vi "MAIN - PECT - Autonics - Pulses.vi"() -> ()   [LabVIEW 2018]
uses:
  Control 1.ctl
  <vilib>/DAQmx/read.llb/DAQmx Read (Counter U32 1Chan 1Samp).vi
  <vilib>/DAQmx/write.llb/DAQmx Write (Analog 1D Wfm NChan NSamp).vi
  <vilib>/DAQmx/read.llb/DAQmx Read (Analog 1D Wfm NChan NSamp).vi
  <vilib>/Instr/_visa.llb/VISA Configure Serial Port (Instr).vi
  <vilib>/DAQmx/create/channels.llb/DAQmx Create Channel (AI-Voltage-Basic).vi
  <vilib>/DAQmx/create/channels.llb/DAQmx Create Channel (CI-Count Edges).vi
  <vilib>/DAQmx/miscellaneous.llb/DAQmx Fill In Error Info.vi
  <vilib>/DAQmx/configure/timing.llb/DAQmx Timing (Sample Clock).vi
  <vilib>/DAQmx/configure/trigger.llb/DAQmx Start Trigger (Digital Edge).vi
  <vilib>/DAQmx/create/channels.llb/DAQmx Create Channel (AO-Voltage-Basic).vi
  Global_data.vi
  <vilib>/express/express analysis/Spectral/Block/exnSpectralBlock spectral measurements PSD poly.vi
  <vilib>/express/express analysis/Spectral/Block/exnSpectralBlock spectral measurements PSD WFM.vi
  <vilib>/express/express analysis/Spectral/XNode/ExpressSpectralMeasurementsBlockNode.xnode
  <resource>/objmgr/daqmx.rc
  <vilib>/Platform/NI_3dgraph.lvlib
panel:
  out "x <= y?":bool
  in  "Motor counter":tag="Dev3/ctr0"
  in  "Motor Counter Terminal":tag="PFI8"
  out "dy":dbl[][](array[numeric])=[[0.02185273217949213, 0.22162137391350623, 0.3780063347527216, 0.47366728119120083, 0.5155987387622605, 0.5344849660156372, 0.5340327156552669, 0.5179164395979683, 0.4924534388561326, 0.4657014009743683, 0.4395619065458265, 0.41345477245652273, 0.38299660763801213, 0.35485913243808975, 0.32430442308230173, 0.30445032009464046, 0.27550721525097666, 0.251882180054519, 0.23418758796048045, 0.2142368598869009, 0.19357706032981925, 0.1801369179101573, 0.1648273984200661, 0.15686645912775665, 0.13830164031007763, 0.12063927272359809, 0.11206594020999994, 0.10861727814154509, 0.09356558004140059, 0.0861847728629872, 0.07722466077804135, 0.07770813065864868, 0.0689091681320213, 0.06265642589408449, 0.055372300069219005, 0.052600467323083766, 0.0475402553312021, 0.041770966987191294, 0.037323135461628354, 0.039031364875901975, 0.03471245509778598, 0.03148938809455126, 0.028782011620806625, 0.02665478726769166, 0.026268020417924642, 0.021852415607831688, 0.014922815304144965, 0.020015267194226194, 0.01804919503626312, 0.01572858483151185, 0.014568279890680547, 0.01592197018079, 0.018564888990501682, 0.01208651666644922, 0.006156065869896921, 0.008379985211604435, 0.012924516058780533, 0.006703988431595143, 0.006865142169170113, 0.005285837275303962, 0.011377442504307389, 0.008412216926839022, 0.006220528313659379, 0.006800681356610383, 0.0037065325418499384, 0.005801529216698853, 0.0029329953769190453, 0.0017726895292300426, 0.006639528072359013, 0.006188298098165568, 0.002997456934826559, 0.0038354556699644604, 0.004673454442502667, 0.005124684635743115, 0.0007735372999029266, -0.00029007654728996357, 0.0031263799247724933, 0.003996609454210542, 0.0011925366909029123, 0.0018693819072517215, 0.0036098409046472213, 0.008122142002352284, 0.0008702294956277612, -0.001095844667359458, -0.001418151804670309, 0.0045445320082038165, 0.0010313830870058993, 0.0007413066156765069, -0.0022239198542619576, 0.008379987983489379, 0.0013536903608795114, -0.0002578458337252343, 0.0016115362047441906, 0.001901612692167376, -0.0004834608665751361, 0.0008379988404314531, -0.0008702295433602458, 0.003319764541380721, 0.0022239199677400734, 0.0014503825811269522, -0.0015148440421395293, 0.0035131489465634047, 0.0017404591631580146, -0.0021594585229163243, -0.0020627664120063116, 0.0014503825799989656, 0.0022883814364993427, 0.002030535662503219, -0.001063613882371861, 0.0025462272945091513, 0.007155221045837656, -0.0023206122806760376, -0.002771842462127694, -0.00077353738382957, -0.00022561499425499676, 0.0016759976704383561, 0.0009669217607966019, -0.004608993606950662, 0.0077676047046848495, 0.0011925368038836481, -0.0016115363216133716, 0.0007413066839978555, 0.0002578458568640585, -0.00035453803645157933, -0.00273961161100722, 0.0020305356825334187, 0.0021594585699595825, 0.0021272279138271344, -0.0003223072593838694, -0.0014503826419236532, 0.002900765285667184, 0.0005801531028586382, -0.0023528429885493196, -0.0019660742882070537, 0.00032230723191783994, 0.002385073698162543, 0.0020305357420138392, -0.0010313832066026762, 0.0011925368768670452, 0.008057681666933547, -0.003964379420267505, -0.004254455948108138, -0.0006768452007133163, 0.001998305074122797, -0.0017082284897318445, 0.0013859212221971617, -0.0032553032595314946, 0.006123837900990026, -9.669220003782897e-05, -0.0004834609598374229, -0.0012247676106964533, 0.0010958447384830095, -0.0006768452835217431, -0.0022561507887344234, 0.0010636139879691697, 0.004286686496722147, 0.0010958447184945541, 3.22307075428796e-05, -0.002610688825346763, 0.003255303372588614, -0.00029007653819057566, -0.0038676871668865687, -0.0012569982994836693, 0.0027073809723914266, 0.0008379988720914611, 0.001837151388540903, -0.0011603061375105028, 0.00022561513089769392, 0.005350300672845698, -0.0019016129023885497, -0.0032875342027223198, -0.0015470748241881438, 0.0013859212779196994, 9.669220112495935e-05, -0.0008379989032860635, -0.00022561506580132118, 0.004286686619572322, 0.00022561507642038237, -0.0023528431049744114, -0.0006123838295124528, 0.0008379989115052666, -0.0006768452570238281, -0.0020949971695305436, 0.001675997810987262, 0.0032875340175193557, 0.000999152537735526, 9.669215431618028e-05, -0.0019983050408773906, 0.0012569983738517365, 0.0005801530509979003, -0.0033197648624758713, -0.001933843537593738, 0.0023528430139325707, 0.002352843003613714, 3.2230727526005865e-05, 0.0003867687163454647, 0.00019338437490290517, 0.004254456017976693, -0.0032230727316582275, -0.0020949972828692154, -0.0008702296034401868, 0.0013859212870555027, -0.0002900765149931317, 0.0004189994079704107, -0.0018371514061916727, 0.004512301822965803, -0.0007735374888504509, -0.0014503827796508162, -0.0009024603734397729, 0.0011603061884652988, -0.001611536337480679, -0.002159458641943779, 0.0015148441911065902, 0.004770147471044872, -6.446143959504269e-05, -0.00012892292785871007, -0.0019660743144251924, 0.002223920178802352, -0.0020627665501065096, -0.00119253690483756, -0.0020949971905164233, 0.001998305023551694, 0.000837998893217673, 0.0011925368763803235, -0.0009346910904382, 0.002127227990854408, 0.0019660744327474333, -0.0017404593293584014, -0.0027718425051004303, -0.0011603061738929554, 0.0011603061928742164, 3.223074204505849e-05, -0.00019338439914129424, 0.0006123838137348514, 0.0024817660569604882, 0.00012892286886057036, -0.0007090760386532224, -0.000225615129568979, -0.00016115363443436337, -0.0006123837841736091, -0.0024495352188536046, 0.0014826134650398615, 0.0032875340681286502, 0.0008057681913156145, -0.0017082285571126121, -0.0007413066611023922, 0.0020627665464481026, -0.000999152585484886, -0.002256150873965801, -0.012408829591370463, -0.021433432067929914, -0.22197293874851098, -0.3764222806586943, -0.46740915295030705, -0.5164638338272902, -0.5334490578309308, -0.5352859904035077, -0.5179780628156556, -0.4965124995471779, -0.46740836721638884, -0.4402703575389572, -0.41110184791818216, -0.3806441179057998, -0.35328052056021786, -0.3275928987712948, -0.3012284032192838, -0.2752506398248955, -0.25397853054603514, -0.23493031326555158, -0.21491513953837904, -0.1958023955316519, -0.17643177172610525, -0.16411968228431473, -0.15132410993446976, -0.13846405632706293, -0.1227998907450889, -0.11590252592732764, -0.10665229070022342, -0.09727311992830856, -0.08679808396375766, -0.08019075848337298, -0.07368011952376108, -0.06742732255462158, -0.06049766823168046, -0.05608203042605808, -0.053213480482009246, -0.0475730563911565, -0.043705337617349294, -0.04022438977457732, -0.037935990066018555, -0.03374595466774899, -0.030458387820377908, -0.028621219564915812, -0.026203890291860432, -0.025752658006232387, -0.019467593462318078, -0.01927420876953434, -0.02078907336652236, -0.020176684123793365, -0.015567634743558045, -0.013246994438153692, -0.013118070851520613, -0.014407317066149616, -0.013537077661091246, -0.009347030152641267, -0.010668507561701013, -0.009798267022355311, -0.010088347912076578, -0.008090017555329787, -0.007445394773112568, -0.00928257069176297, -0.005092521345138934, -0.0058338382012763645, -0.004125587253031249, -0.00728424031063124, -0.005028059898926074, -0.0032231152560280307, -0.005801607890615124, -0.005092522415750089, -0.005801608187410601, -0.0037065829285172214, -0.002320643368463493, -0.004834673724378291, -0.0028041107197980253, -0.0015148644444460402, -0.00022561814109067768, -0.00409335720323778, -0.00438343776733241, -0.0029974979706475224, -0.0009024725041406612, -0.003384271962996621, -0.002449568288255044, -0.0026751867248657746, 0.0009024725590478511, -0.00286857347007885, -0.0007090853837512512, -0.0033198098144016086, -0.0010958596788803732, -0.0028041112816303837, -0.0018694075623315598, -0.0011603217624793771, 3.223115459860537e-05, -0.00016115582712750154, -0.0013537089395612156, -0.003480965935072966, 0.0026429556728508885, -0.003061960775959882, -0.000870241426966345, -0.004737981658807122, 0.0011925533678454059, -0.0014826337024933522, -0.00038677395914277213, -0.001933870000138782, 0.0021594881681208378, 0.0010636284382137262, -0.001998332242745704, -0.002836342690361704, -0.002965267523460824, 0.001321477918626357, -0.00025784932654815407, -0.003287579153148812, -3.223132886898128e-05, 0.0026107244517081796, -0.00012892453675217297, -0.0013859400535904953, -0.0014504025112538343, -6.4462473896576e-05, -0.0030941922480201, -0.0012247844018435927, -0.00016115567855923274, 0.002127257150072559, 0.0013537090959196973, -0.0016760207747053002, -0.0017082520566722437, 0.0023206442516912063, -0.002127257163786034, -0.0019983324466084085, -0.0012570157816984562, -0.0010958596522536723, 0.0020627948594293954, 0.000419005267335848, -0.002900805281237595, 0.002739649366902519, 0.0035454285251645956, -0.00438343887530479, -0.0011280909248192472, -0.003061961217107445, 0.0024495689780037466, -3.223119648865236e-05, -0.0016760208118133946, -0.0010636287683363221, 0.0033520414134819987, -0.0004190049852823563, -0.0026429558725240554, -0.0011925531630785358, 0.0015470960247538912, -0.0027074183199484736, -0.001289246809195177, 0.00128924691794019, 0.002610724760119254, 0.001901639043667025, -0.0030941922624947438, -0.0032231171698793304, 0.0060272289191773964, -0.004931368989611329, -0.0008702416052575046, -0.0019016393047914804, 0.0020305639428972455, 0.0012892468470901974, 0.0006446234421115804, -0.002610724837572853, 0.0019016390284969376, 0.0015793272920747725, -0.0017082519598439205, -0.002900805364877357, -0.000709085817734767, 0.0028041119282748994, -0.00016115587107901064, -0.0018049455564170813, 0.00022561808799004268, 0.0013537090055955048, 0.0008380105330507703, -0.003255348141158798, -0.00035454279478663864, 0.0018371766375260279, -0.0035776600751207255, -0.0004190052285268919, 0.002900805448792454, 0.002223950819624676, 0.0018694079109380368, -0.0032553481382180394, -0.0032875795671039043, 0.004447901674611288, -0.0025784936590147467, -0.0016115585622911155, -0.002127257495139645, 0.003255348419116011, 0.0018371768337592798, -0.001128090974523488, -0.0009669351580914309, 0.0009024727918127695, 0.001128090987530861, -0.0025140313757301413, -0.0011603221493157179, -0.0009669351707461971, 0.0036743535752394862, -0.0016437897422942882, -0.00016115587246545715, -0.0003867741019458748, 0.00077354797094209, 0.0001289246734081928, -0.0019338701466384833, -0.0028363430810758317, 0.004351208139382834, -0.003029730220318605, -0.00048346763104412105, 0.0020627950775606863, 0.004415670395760962, 0.0001933871398263065, -0.0042867457023128, -0.0020305639252988783, 0.004351208217657998, -0.0028685742179446194, -0.000966935188323248, -0.003932203230262665, 0.005833842290003943, 0.001676021002762873, -0.0002578493208744703, -0.0023528755324573325, 0.0001933869506860475, -0.0015793273811111064, 0.0009024727892432693, -0.0025784937121944296, 0.0008057793101148292, 0.005608223865920969, -0.0019983326508024035, -0.0013859403391727199, 0.0009991662564088344, 0.000386773835537646, -0.0011280909016528895, -0.0028685742308987017, -0.001063628580464382, 0.0019016390821331441, 0.000451236446354919, -0.0012247846328268253, 0.002127257322039, 0.005060293783419212, -0.0009347038394702523, -0.005350374306660299, -0.000322311809180853, 0.00228841316574524, -0.0023528754941306573, -0.0006446235024473168, -0.0026751874774042506, 0.005092525334164044, 0.004028896469372434, -0.004770213274351676, -0.0007413169580825496, 0.0015470961610528633], [0.026784100031834512, 0.22565025518823933, 0.3745898180588192, 0.4658351284321114, 0.5195309092491112, 0.5352584960489501, 0.5372235546955544, 0.5137586578368909, 0.49219558678815245, 0.4708260749714661, 0.4421403513412341, 0.41177877159702825, 0.37458440957515166, 0.35463351738372256, 0.3285910937384298, 0.29984134272168944, 0.27844020024186034, 0.24917480927999724, 0.2327049801329557, 0.21581615988325065, 0.19805711606493515, 0.1764948588357853, 0.15873581094289735, 0.15038810220007237, 0.13901071275952415, 0.12424910299364411, 0.11619146185751328, 0.09917369791631492, 0.09872248304086018, 0.08898883938039681, 0.08389640742510363, 0.0708752299975064, 0.0624952645947654, 0.06462249593467728, 0.058144137574782206, 0.054566538291412225, 0.0439304186397127, 0.04270565633641521, 0.04160981659824259, 0.03767767582517134, 0.03825783118913595, 0.02359286790303816, 0.027911782375556804, 0.02868532082928832, 0.025268868363350627, 0.02265818289102217, 0.016276504724094476, 0.019112807239303642, 0.01946734585367027, 0.016340968153478297, 0.01701781357957932, 0.0065428338386475104, 0.012924514293859879, 0.015019510914417111, 0.011280748870691415, 0.010990672788820266, 0.005865989716593134, 0.010700596721945121, 0.010700597051142235, 0.01024936728566983, 0.00667175803059461, 0.0016759972379327692, 0.00818660189065934, 0.007993217768344607, 0.009443600123263174, -2.8045121780451154e-11, 0.0060271442455350765, 0.006317220804501922, 0.005092453598039448, 0.0069940660319938175, -0.0012247673040803875, 0.0008057679314195099, 0.004770146517182106, 0.006381682601488414, 0.004318916540771767, -0.0033519948913074415, 0.003642071348493481, 0.004028840109692844, 0.0029007649154300097, 0.003319764295098615, -0.0015148438851326773, -0.0002900765221385271, 0.004061070905809316, 0.0037065330108747574, 0.002707380653014013, -0.0028685342311973727, 0.003835455906583185, 0.005124684906207655, 0.003609840897486727, -6.446145531402436e-05, -0.0012569981537113861, 0.001514844018148942, 0.0026429193096486614, 0.006671759686645906, -0.002578457828548153, -0.0015793054971009468, 0.004061071147166473, 0.002256150657456324, 0.003577610328740377, -0.006381683273562366, 0.0024173042075394946, -0.000870229533275868, 0.004802377867471286, 0.0023850735957813285, -0.005285838697146161, 0.0006446144220459971, 0.0019016127094797497, 0.0022239199659042086, 0.0029007652016312946, -0.0067039906215544676, 0.0017404590713407941, 0.00141815186330696, 0.0037387640277160017, 0.0012892289743620111, -0.0028685344298740034, -3.223070115243587e-05, 0.004093302016091371, 0.0042866863703157065, -0.0008057681690694096, -0.0038999176292229265, 0.00344868754693195, -0.0012247675085372833, 0.006220529854120471, -0.0020949970438994825, -0.0013536905259066145, -0.0006446144910023932, 0.0038354563162972255, 0.0021594585312509906, -0.00554368468580968, 0.0005156915346216095, 9.669218883434638e-05, 0.0022883814829333105, 0.003255303272983845, -0.005350300361256721, 0.0014181518631035672, -0.0010636139326178906, 0.0034486875947035145, 0.0018693821012547573, -0.005414761836013859, -0.0006123838185558839, 0.0022883815314544975, 0.0034164568482051294, 0.0008379988633855362, -0.002385073645239544, -9.669216226537714e-05, 9.669221445562926e-05, 0.006736221596612246, -0.0014826134029650717, -0.0034809183239419283, -3.223075455771607e-05, 0.0033519955214398323, 0.0043511479505315975, -0.0024495351252111774, -0.00032230729171445205, -0.003384226219839803, 0.0027396117090177086, 0.004093302137440524, -0.006478375868526065, 0.0016115362569033564, -0.004383378652741854, 0.006542837273798341, 0.0008057681411504092, -0.002320612220817253, -0.0005156916361865882, -0.0026751502307664765, 0.002513996586062106, 0.0010313832376551701, -0.0016115362806203848, -0.0021272278927808586, 0.0005156916355364416, 0.005994914960246511, -0.00038676870819553955, -0.0013859211626288115, -0.0018371514158426194, 0.0015148442178105626, 0.002900765255988702, 0.0007090759568981753, -0.0022561508063683178, -0.0017404592034209188, 0.002449535187906804, 0.005640377065394553, -0.0033842261968022314, -0.0005479223863940064, -0.004157763665022962, 0.003964379299580045, -3.223077380098971e-05, -0.0020949971808610357, 0.0007090759662649049, -0.00364207199467792, 0.0044478401379102195, 0.0017726899490213555, -0.001998305021256641, -0.001224767571348373, -0.0013214597760997648, 0.002449535171817452, -0.0011280754215361455, 0.0011280754242681823, -0.0038676871074336816, 0.002191689378442163, 0.003351995498111826, 0.0017082285051648327, -0.0016759977555693695, -0.002997457540887538, 0.0016759978047211632, 0.001901612802326369, 0.0005156915794106709, -0.0006123837798819309, -0.0024173044457338477, 0.003706533509498122, 0.0014503826651166563, 0.00041899950810631026, -0.0022239201605689374, -0.003351995526546858, 0.002094997185965397, 0.000934691034405688, -0.0025462273575529437, 0.0010636139657895782, -0.003384226213441366, 0.0038676870960570042, 0.0007735374273947215, 0.0017404592379204331, -0.004834608930694095, -0.0011603061501794798, 0.004286686585561306, -0.002513996664216478, 0.001966074317046207, -0.0030941497023038167, 0.0013859212261548848, 0.002868534653052812, 0.0006446145146608018, 0.002417304477217108, -0.005898222917110729, 0.002642919582378944, 0.0005479223307247594, 0.002062766444883124, -0.0019983050164809057, -0.001675997733743273, 0.0028040731655680773, 0.0015148441303747262, 3.2230793463483565e-05, -0.0004834609410648838, -0.004157763717199892, 0.0009991525044208416, 0.0007735374197315181, 0.0002900765379800774, -0.0023850737280328715, -0.0019660742776830276, 0.003609841311993378, 0.00019338434379356784, -0.009701448515547106, -0.023335044661842552, -0.22706538836152435, -0.37313474393759405, -0.46892398895940657, -0.5155936015835576, -0.5403141757711412, -0.5309348546694241, -0.5150450772119163, -0.49367620674724616, -0.46666706394703106, -0.4418174290863563, -0.41016716126580566, -0.38006396776770957, -0.35144337261062875, -0.32772182213135537, -0.30361347886788836, -0.273864719257253, -0.25207691524432363, -0.23154607781170622, -0.21494736791704883, -0.19776847544427945, -0.17930031899887577, -0.16218582922158253, -0.14881009816772917, -0.13959213730365772, -0.12844030616179314, -0.11119680656945619, -0.10391265692273333, -0.0949202558992468, -0.08873194194834788, -0.08096430144458733, -0.07219749111723939, -0.06694385552970061, -0.060304280391832776, -0.059272903571049085, -0.0533746352299751, -0.0436730962504015, -0.04138469878758588, -0.03993430829718658, -0.03851614811812887, -0.033133562469370936, -0.030684004278646704, -0.027879902850996174, -0.02659066240223673, -0.026042736991306548, -0.024721264573471124, -0.015696554150562037, -0.018855205388085494, -0.018855207112675743, -0.019532062584926457, -0.014858550554825989, -0.012408985582960774, -0.01398831198034678, -0.011055279609098356, -0.015051941356329479, -0.009250337089361516, -0.005866067654448415, -0.009218106689512062, -0.007606549910546434, -0.012892458165605802, -0.002288411469471896, -0.0071230835353617294, -0.007413164173106779, -0.0048991348009987945, -0.009024722272534369, -0.002385105232974638, -0.002868572547725101, -0.0025784921129536897, -0.006091687985520622, -0.007445396686291517, -0.00022561813226662508, -0.004383437116983302, -0.0031586533755119106, -0.0055437589730216175, -0.005189216411267239, 0.0006446231927963453, -0.0023528745689338493, -0.0023528745728080835, -0.005060291990865551, -0.005866071164223996, 0.00299749793514259, -0.0044156689913359415, -0.00048346743909188916, -0.005189217061991158, -0.0009347036610325432, 0.0008057790414079946, -0.0007090854953375469, -0.0012247841912307322, -0.005898302776362385, 3.2231152168549215e-05, 0.0010313972178455089, -0.0020950256319416383, -0.0009991661126473872, -0.004318976020729615, 0.0012570153559829933, -0.0013537088386508245, 0.0035454280963973517, -0.00409335779920017, -0.0032875788193740263, 0.0007735479510762033, 0.0003545428644864401, -0.00041900529834837386, -0.003448734694744715, -0.003319809998934886, 0.0024173375156335553, -0.0014504024769417256, 2.567546175669122e-11, -0.002836342661311164, -0.0033842724971959726, 0.0012570155493758506, 0.0012247843204322706, -0.0007413168383001434, -0.003416503759653189, 0.00019338705136906498, 0.0013537090238626703, -0.0016115583255649213, 0.0025462621815215414, -0.005769378940321701, 9.669348670282574e-05, 0.0018694076644338864, 0.0030297297316268512, -0.0018371765356848258, -0.0031264232430725514, 0.0005479298020878431, 0.0004190052097685637, 0.000838010392544497, -0.0019016388201507084, -0.002127257114010739, 0.0005801610183748807, -0.0001611558044478656, 0.002997498480917571, -0.004802444044615051, -0.0019661012238030295, 0.0014826338573845632, 0.0005156986527428131, -0.0014826337252324961, -0.002642955856408946, -0.0018049454808322096, 0.00283634286599721, -3.223118070128095e-05, 0.003126423335084283, -0.005447067514157133, -0.0009347038785447737, 0.0030297298815264995, 3.796962744218035e-12, 0.0007090857046625487, -0.0028685740616705147, -0.000999166267717122, 0.003255348036048211, 0.001708251938849159, -6.446229686307703e-05, -0.0030619610776065898, -0.0009991661907848837, 0.0015470961224055557, 0.001998332483110765, -0.0033520415490624345, -0.0014504026452346608, 0.0003223117461077507, 0.0020305636674180505, 0.0004190050384522692, -0.0005479298540107536, -0.004447901330258297, -9.669342538742853e-05, 0.0009669350817098632, -0.0005156987385133149, -0.002062794903411991, -0.0008380103899510161, 0.0016437896337384572, 0.0011280908943396284, 0.0008380104467677896, -0.0014181714313679095, -0.0028363429613520452, 0.0053826053679344454, -0.001966101330236114, 0.0018049454987920655, -0.003513197568158155, -0.0005156987394574486, 0.003061961127403201, 0.0015148649466905084, -0.0008380104064142913, -0.0022884130471547692, -0.0009669350511911645, 0.0027718806427072806, 0.0014826337522340083, -0.0024173376503648925, -0.0038677405154965427, 0.0006768546838422651, 0.0016115585356173412, 0.0008702414517678392, -0.0013214779622430228, -0.00157932726729193, -0.00174048317656883, 0.001289246833080071, 0.0012570156056801451, -0.0021594884768356692, -0.0032875793745299475, 0.003835509306993501, -0.00012892477700532368, 0.002642956048963363, -0.002320644239499181, -0.0015793273909219252, 0.002191719609478504, 0.0008702415896912896, 0.0030941923712584085, -0.004576826281601498, -0.002514031285067553, 0.004673519766448031, 0.0007413167925802711, 0.0012570156416025213, -0.004286745550196258, 0.0005801611322269196, 0.002159488395125919, 0.00025784929858208017, -0.0011280908768931397, -0.0046090574176513854, -0.0007735480921899907, 0.0046412886076723225, 0.000838010401848166, -0.0018694078646959156, -0.0041255899279191155, 0.0021594885187861124, -0.00032231168083995954, 0.002933036524756183, -0.0017082520723921135, -0.00448013281349624, 0.0014181715104699677, 0.002933036480482265, 0.0030297300803647786, -0.0017082519297382248, -0.004028896421838013, 0.004866906803883353, -0.0011925534246222114, 0.004737982080823322, -0.00451236385494358, -0.002127257225150281, 0.0021917196301046715, 0.0008702414624286448, 0.002965267697288887, -0.0058338417378269725, -0.0011280909005098039, 0.004480132621861088, -0.0007735480983974696, -0.0009024727385416043, -0.0027074184294688663, -0.0023851065415758654, 0.0023206443362235873, 0.0030941924315275315, -0.0014181715573906573, -0.0036098912108366576], [0.023722137762525186, 0.2371245241325024, 0.38622519292709967, 0.481757169166837, 0.5292323109001864, 0.54653917824941, 0.5429282811959335, 0.5240723850532003, 0.5014456946514636, 0.4697623674048248, 0.4458790338310945, 0.41158533032513056, 0.3851882435479477, 0.3508947345990861, 0.32710846668232973, 0.2997768719803513, 0.27576505771064386, 0.25172103035887816, 0.22893400647220252, 0.21165842138200297, 0.19103085385029006, 0.1789443985045689, 0.1602184331582115, 0.14655267156696095, 0.13424059275309386, 0.1217351260244528, 0.11283948730191895, 0.09891586380494255, 0.09346889761880117, 0.08176918147313206, 0.08051219657246023, 0.06939262671702551, 0.06578279984400393, 0.05733837042176759, 0.05501776763805788, 0.04882948224765338, 0.044059345414734, 0.040739588374155034, 0.035840526695137154, 0.03706529570758432, 0.03023239108652609, 0.030780314901592387, 0.025462251500319333, 0.02481763888330013, 0.02414079550206738, 0.020240881535092292, 0.01985411402224546, 0.013665819214494057, 0.017597965985173936, 0.012312130421926248, 0.01879050337970245, 0.010249365860009352, 0.011796440173688527, 0.010410519911922655, 0.01121628795723062, 0.010023751843414974, 0.007896524957960338, 0.008347755055396089, 0.00422222371416936, 0.00867006247417379, 0.006059374640241089, 0.007735371980243322, 0.004544531098360949, 0.004931299781560483, 0.006413912835881774, 0.002030535274879064, 0.0053825299953356165, 0.0021594581464041696, 0.007026296790251685, 0.0011925366345426625, 0.004512300782119283, 0.002417303936651294, 0.003996609292132192, 0.0042866858269237085, 0.0025462269272100713, 0.0007090758506471673, -9.669215711749501e-05, 0.0031586106657695012, 0.0007090758525132301, 0.0049957618120464176, 0.001160306047379045, 0.0015793053023820391, 0.0008379987777615838, 0.0020627661903942496, 0.005382530604197022, -0.0012892288849890576, 0.002836303552124164, -0.003770994492832358, 0.004254455360038101, -3.223069782709587e-05, 0.0034486872793451084, 0.00125699822586256, 0.0013536903546604862, -0.00035453797070594817, 0.001031383154003862, 0.0008702295405598193, -0.0009346909913015011, 0.0043189169383826, -0.0013214595822379493, 0.001579305409647347, 6.446141937299643e-05, 0.0013536903620590124, 0.004318917010436962, -0.001708228395968625, 0.0011280753208140482, -0.004415609122220943, 0.0038032253786566272, -0.0010958446210613815, 0.003932148327610463, -0.001095844513787192, 0.0009991523456758244, -0.0010313831854258382, 0.002900765191198751, 0.0024495350416895434, -0.001869382006516318, 0.0016437669033235736, -0.0042222248437528975, 0.004157763422337979, -0.00019338432674675943, 0.0007735373470447726, 0.002320612203359218, -0.0009024602962526274, 0.0013859211266735727, -0.0013214596983965876, 0.002062766381802028, -0.003094149570099347, 0.004608993638596459, -0.0028363037173066985, 0.002417304350713856, -0.0021594586044884068, 0.0028363037586780493, 0.0028040730936726987, -0.0020627664154995173, 0.0012892289769519394, -0.004157763495366673, 0.0023528428979586735, 0.0004189994073700021, 0.0015148440748324887, 0.00019338447650696367, -0.00019338443107130843, -0.00106361397243937, 0.0022883815140222197, 0.003706533412026758, -0.002771842382415457, 0.0013859211452835751, -0.005962684099082516, 0.0050602238125820875, -0.001837151306567364, 0.002062766369500757, -0.0009346909577585549, 0.0005801530509703667, 0.0007413066153727499, -0.0005156915862318812, 0.0011925368322467378, -0.0021916893096429746, 0.0017726898802443714, -0.0009669216916297074, 0.0025139965711895584, -0.0028363038495680115, 0.0013536903976367753, 0.003996610004563195, -0.0028040731106164785, 0.0008702295343994138, -0.005027993118993379, 0.0033197646849512097, -0.0007413067025794362, 0.002836303834905074, -3.223059878365575e-05, -0.001160306205127526, -0.0013859212242408603, 0.0024817658828464317, 0.0022239200809721638, -0.0011925368656120483, 0.000644614465025839, -0.004576762960862624, 0.003964379203323709, -0.0017404591520797652, 0.0015470747938852725, 0.0006123838738565368, -0.0027718424539182607, 0.003642071964934601, -0.0023206122339409774, 0.0015148441139851698, -0.001675997748059821, 0.0030619189209630804, -0.002449535063711039, 0.0024817658408915477, -0.0019983049961789234, 0.0009346909881626786, 0.0017404592536793828, -0.0010313832079944518, 0.0010958446014051049, -0.004995762439449436, 0.0029652267256548015, -0.0005156916062691863, 0.001837151341817389, 0.000128923018110072, -0.0009024603769702821, -0.0007735374634521008, -0.0003223072499665136, 0.0037065335087183016, -0.00022561509067919872, -0.00025784586254040676, -0.004963531711946523, 0.006059376394000893, -0.0028040731371392624, 0.001966074260496775, -0.0008057680093491726, -0.0017082285522711516, 0.00022561505178320118, -0.00022561508596119495, 0.0010958446957829437, -0.0008057681547803952, 0.0014503826727061409, -0.0006123837254952136, 0.0006446144683875943, -0.0009991525112260646, 0.000547922299396042, 0.0024817659713631812, -0.0026751502593853616, 0.0015793055151691604, -0.005092454627643406, 0.004286686488092606, -0.0023206122626335812, 0.004383378691879436, -0.00048346073530325384, -0.002256150872242735, -0.0002900765921323156, 0.0012247675802248281, 0.0013214598240773867, 3.2230729531512736e-05, -0.00029007661669844254, -0.004608993751203272, 0.0037387641329704735, 0.0005479223477546924, 0.0009024603267882014, -0.0009669216550065585, -0.002159458687792437, 0.0019660742175870993, -0.0029974574763578232, 0.0029007652828862973, -0.0008057681395543526, 0.0026106887979988613, -0.002127227832978029, 0.002642919478063277, -0.001675997763636694, 0.001708228452548255, 0.0009346911229579646, -0.0020627664732550954, -0.011731984088416247, -0.030135726704125787, -0.2260339980030075, -0.38960461090200704, -0.47927000398948394, -0.5281312886793872, -0.5498866417693702, -0.5421833196456392, -0.5247464862755081, -0.4987041952347353, -0.47491813219753365, -0.44242985659381673, -0.4168711938981533, -0.37793681069863605, -0.3535062092717087, -0.3233062900484449, -0.3022598635971412, -0.2771845630346572, -0.25159352884923836, -0.2317073055320189, -0.20811450076104565, -0.19428760671142387, -0.17385335800030655, -0.16170241789188378, -0.14694075352827296, -0.13266253056405075, -0.12134953492685785, -0.11135799381862466, -0.10384822584913245, -0.09134264317759921, -0.09044021163799254, -0.07274541407064383, -0.07200412430742986, -0.06098113020870333, -0.059820829725975244, -0.055211803988806096, -0.05021600250734881, -0.043608643548181725, -0.03925745652707491, -0.03803268235150803, -0.036582289932793444, -0.03561536374969876, -0.02427002050400162, -0.025752654579044965, -0.02275516429528235, -0.024270029681635386, -0.022787400624052268, -0.017533730125073532, -0.020853537824341295, -0.011570974778586596, -0.01949983365297836, -0.011732132246434546, -0.011699902039092436, -0.010249501230262581, -0.011828827667042852, -0.00838009632204706, -0.00979826710285181, -0.010571814869559049, -0.006671846916394664, -0.011248669926010813, -0.003932199812865633, -0.0075098575572773996, -0.0037710444655205677, -0.005704913678328261, -0.006704079249814754, -0.0038677382299674434, -0.005704914019310614, -0.001804944583051693, -0.005704914238438441, -0.0035776580879129938, -0.007413165820525869, 0.001353708604491466, -0.003964432172964827, 0.001031396934382478, -0.007703246804886987, -0.0024495678157681056, -0.0005156983666481096, -0.006414000593433222, 0.0021594876372166283, -0.004770211566744287, -0.0007090855330753598, -0.0021917189942461945, -0.00029008034253763526, -0.0014181710537481962, -0.002191718855028668, -0.0002900805702168441, -0.003513196579267408, -0.00022561810969357055, -0.007284242673396335, 0.0032231163898037707, -0.003932201882808073, 0.0028685734701046073, -0.0017404828591658372, -0.0012892464315834573, -0.0023851061566340093, -0.0012247841201391552, 0.002739648844661602, -0.0018694076149685657, -0.0029008046919942743, -0.003996664253230087, 0.0018694076316334574, -0.0007735480160491193, 0.002965267061536103, -0.003448734685068011, -0.0027718800567431146, 0.0009024727253645892, -0.0035131970128698953, 0.0034165035179638537, -0.004576825464208234, 0.0027396490691682374, -0.0031586543805905976, 0.002159488243041352, -0.0013537089425170734, 0.0006123921473211169, 0.00029008041550859787, -0.003029729612078036, 0.0008702415731836055, -0.005447067100965874, 0.0026751868466918793, -0.0017404829650056186, 0.0028363425996262848, -0.0007413169714398649, -0.0030297295485715026, 0.000805779057329481, -0.0012570153434090514, 0.0034487347782690136, -0.0021917194071248147, -0.00012892465011038468, -0.005285911296502022, 0.003061960958957499, 0.0008702413947840881, 0.0015793272198170172, -0.0024495688385481884, -0.0018694076230119094, -0.00016115573398778338, -0.0005479298334014615, 0.0031264232173411344, -0.004254514104774287, 0.0018371765618727665, -0.0022884130342184505, 0.0006446234765116188, 0.002610724601320058, -0.0017404830309395436, 0.002095025768024783, -0.0039322024231562835, 0.0012570156228823848, -0.004254514192360226, 0.0035131973847049025, -0.0033842726588177996, 0.003384272645244657, -0.001095859882928707, -0.002191719305275619, 0.0017082518590303408, -0.0018694076790159997, 0.0033198102900460214, -0.0009669351749996835, -0.0007090856304134974, -0.004222282986558135, 0.0025784935561627975, 0.0019338699521185276, 0.00022561828239631154, -0.002256181897001497, -0.00222395066343406, 0.0030941922295824043, -0.003255347905323447, 0.004544594746034747, -0.004125589663886764, 0.0017082520191262773, -0.001579327332937197, 0.0008702416187382767, 0.0010313974397924142, -0.00022561817276489649, 0.0009347037804072755, -0.002352875254761244, 0.0012892467869516366, -0.003287579223941961, 0.002417337682913079, -0.0017082519186955025, 0.0015148649436582673, 0.00041900501455138794, -0.0032553478768679867, 0.0019983324096068955, -0.003029729815290594, 0.005414836294768577, -0.0027718805021228476, 0.00048346753665118314, -0.002900805155865882, 0.001998332520356527, -0.00019338709075356064, 0.0023851065162832086, -0.002062794907236487, -0.0032553480007369018, 0.0023206441377405795, -0.0021594882234214907, 0.00386774025704284, -0.0025140312264060327, 0.0009024727373514452, -0.0012570156746782857, 6.44624198162802e-05, 0.0017727143283465807, -0.0014826337528184297, 0.0020950258335776795, -0.003158654481786094, 0.0026107246994797606, -0.004157820793504463, 0.003416503942670346, -0.0029008052157779574, 0.0024818000417710095, 0.0001289246388607168, -0.0022239505987275976, 0.0008380103409475481, -0.0018694077929737318, 0.004512363627270588, -0.0017404831115932495, 0.00029008051913503863, -0.0015470960856358573, 9.669355971020366e-05, 0.0022239506172994083, 0.00041900518009985177, -0.0006446234015022867, -0.004093358497596178, 0.0019983325145398467, -0.0007735480600103983, 0.002868574067686147, -0.0021917195238936316, 0.0007413169026388999, -0.001804945470972541, 0.0006768545709086027, -9.669346880070151e-05, 0.00012892467491809612, 0.0006768544534541121, -0.002868574012261149, 0.0036421221008255955, -0.0027074181727870794, 0.001547096073413634, -0.0016760207959229945, 0.001514865031140289, 0.0004834674826055263, -0.0011925531980692128, 0.00012892462539237926, -0.0032875792495863365, 0.004609057206292455, -0.002320644184202969, 0.0017082520003341983, -0.0018049455434647754, 0.0012892468522887057, 0.0011603220625673316, 0.0003223116747594901, -0.0003223116762312017, -0.0029330364474153825]]
  in  "2D Array In":dbl[][](array[numeric])
  out "Output":dbl[][](array[numeric])=[[0.3400814353200291, 0.34085307883176075, 0.339830570171676, 0.0, 0.0, 0.0, 0.0, 0.0, 0.0, 0.0, 0.0, 0.0, 0.0, 0.0, 0.0, 0.0, 0.0, 0.0, 0.0, 0.0, 0.0], [0.3406381630641981, 0.3402773147220812, 0.34024178819671697, 0.0, 0.0, 0.0, 0.0, 0.0, 0.0, 0.0, 0.0, 0.0, 0.0, 0.0, 0.0, 0.0, 0.0, 0.0, 0.0, 0.0, 0.0], [0.34050743091577346, 0.34047529550682004, 0.34019899894778577, 0.0, 0.0, 0.0, 0.0, 0.0, 0.0, 0.0, 0.0, 0.0, 0.0, 0.0, 0.0, 0.0, 0.0, 0.0, 0.0, 0.0, 0.0], [0.3403223891147707, 0.3401714122724132, 0.33965894768004534, 0.0, 0.0, 0.0, 0.0, 0.0, 0.0, 0.0, 0.0, 0.0, 0.0, 0.0, 0.0, 0.0, 0.0, 0.0, 0.0, 0.0, 0.0], [0.34031088455167346, 0.3403376971894986, 0.3403051870590302, 0.0, 0.0, 0.0, 0.0, 0.0, 0.0, 0.0, 0.0, 0.0, 0.0, 0.0, 0.0, 0.0, 0.0, 0.0, 0.0, 0.0, 0.0], [0.33994324900970335, 0.33976666107566045, 0.34025315048538757, 0.0, 0.0, 0.0, 0.0, 0.0, 0.0, 0.0, 0.0, 0.0, 0.0, 0.0, 0.0, 0.0, 0.0, 0.0, 0.0, 0.0, 0.0], [0.34044597061858256, 0.3406911878474111, 0.34071019609916225, 0.0, 0.0, 0.0, 0.0, 0.0, 0.0, 0.0, 0.0, 0.0, 0.0, 0.0, 0.0, 0.0, 0.0, 0.0, 0.0, 0.0, 0.0], [0.34013462135361405, 0.34017572507322086, 0.0, 0.0, 0.0, 0.0, 0.0, 0.0, 0.0, 0.0, 0.0, 0.0, 0.0, 0.0, 0.0, 0.0, 0.0, 0.0, 0.0, 0.0, 0.0], [0.34090395783956673, 0.3404385025448228, 0.0, 0.0, 0.0, 0.0, 0.0, 0.0, 0.0, 0.0, 0.0, 0.0, 0.0, 0.0, 0.0, 0.0, 0.0, 0.0, 0.0, 0.0, 0.0], [0.33983291330384324, 0.3400365719504464, 0.0, 0.0, 0.0, 0.0, 0.0, 0.0, 0.0, 0.0, 0.0, 0.0, 0.0, 0.0, 0.0, 0.0, 0.0, 0.0, 0.0, 0.0, 0.0], [0.3407806449034506, 0.3402163516722619, 0.0, 0.0, 0.0, 0.0, 0.0, 0.0, 0.0, 0.0, 0.0, 0.0, 0.0, 0.0, 0.0, 0.0, 0.0, 0.0, 0.0, 0.0, 0.0], [0.34052406837097704, 0.34004352845633123, 0.0, 0.0, 0.0, 0.0, 0.0, 0.0, 0.0, 0.0, 0.0, 0.0, 0.0, 0.0, 0.0, 0.0, 0.0, 0.0, 0.0, 0.0, 0.0], [0.33970489509215207, 0.34014077028995776, 0.0, 0.0, 0.0, 0.0, 0.0, 0.0, 0.0, 0.0, 0.0, 0.0, 0.0, 0.0, 0.0, 0.0, 0.0, 0.0, 0.0, 0.0, 0.0], [0.3401809093897732, 0.34017903322060716, 0.0, 0.0, 0.0, 0.0, 0.0, 0.0, 0.0, 0.0, 0.0, 0.0, 0.0, 0.0, 0.0, 0.0, 0.0, 0.0, 0.0, 0.0, 0.0], [0.34040516816508026, 0.34051475253300933, 0.0, 0.0, 0.0, 0.0, 0.0, 0.0, 0.0, 0.0, 0.0, 0.0, 0.0, 0.0, 0.0, 0.0, 0.0, 0.0, 0.0, 0.0, 0.0], [0.34045788854716397, 0.34042044548379247, 0.0, 0.0, 0.0, 0.0, 0.0, 0.0, 0.0, 0.0, 0.0, 0.0, 0.0, 0.0, 0.0, 0.0, 0.0, 0.0, 0.0, 0.0, 0.0], [0.34001362858663825, 0.3402335066009852, 0.0, 0.0, 0.0, 0.0, 0.0, 0.0, 0.0, 0.0, 0.0, 0.0, 0.0, 0.0, 0.0, 0.0, 0.0, 0.0, 0.0, 0.0, 0.0], [0.3401987186221436, 0.34023565108272735, 0.0, 0.0, 0.0, 0.0, 0.0, 0.0, 0.0, 0.0, 0.0, 0.0, 0.0, 0.0, 0.0, 0.0, 0.0, 0.0, 0.0, 0.0, 0.0], [0.3401748767205713, 0.33977270907717305, 0.0, 0.0, 0.0, 0.0, 0.0, 0.0, 0.0, 0.0, 0.0, 0.0, 0.0, 0.0, 0.0, 0.0, 0.0, 0.0, 0.0, 0.0, 0.0], [0.3402474665184202, 0.340495873818771, 0.0, 0.0, 0.0, 0.0, 0.0, 0.0, 0.0, 0.0, 0.0, 0.0, 0.0, 0.0, 0.0, 0.0, 0.0, 0.0, 0.0, 0.0, 0.0]]
  out "Current  Position (mm)":dbl=8.0
  out "Acquire":bool=TRUE
  out "Numeric":dbl=8.0
  out "Enum":T1(ring)
  in  "Direction (+)":string="+"
  in  "Tab Control 3":enum32{"Control", "Data Processing"}(tab)
  in  "Encoder":bool
  in  "Home":bool
  in  "Exit":bool
  in  "Scan":bool
  in  "Move Dis(mm)":dbl=60.0
  in  "Right":bool
  in  "Forward":bool
  in  "Left":bool
  in  "Backward":bool
  in  "Stop":bool
  in  "Pulser Trigger":tag="/Dev3/PFI0"
  in  "Edge":i32(ring)=10280 items=["Rising"=10280, "Falling"=10171]
  in  "2 Plots":bool
  in  "Offset":bool
  in  "Open csv":bool
  in  "Save Scan mode":bool caption="Save Process"
  in  "Gate 1":dbl
  in  "Gate 2":dbl=50.0
  in  "Open tdms":bool
  in  "Tab Control 4":enum32{"Basic", "Gaussian", "Chirp"}(tab)
  in  "Pulse Basic":T3={"Basic amp"=2.0, "Duty cycle %"=50.0, "Basic freq (Hz)"=200, "Basic Type"=2} {"Basic Type" items=["Sine Wave", "Triangle Wave", "Square Wave", "Sawtooth Wave"]; "Duty cycle %" format="%#.2f"; "Basic amp" format="%0.2p"}
  in  "Pulse Gaussian":T4={"Gauss amp"=4.0, "Gauss Nor. Band"=0.5, "Gauss atten (dB)"=6.0, "Gauss freq (Hz)"=1000.0}
  in  "Pulse chirp":T5={"Chirp amp"=2.0, "Chirp f2"=1500.0, "Chirp f1"=500.0} {"Chirp f1" format="%0.2f"; "Chirp f2" format="%0.2f"; "Chirp amp" format="%0.2f"}
  out "Motor Pulse Count":i32=486
  in  "Start idx":i32=140
  in  "End idx":i32=380
  in  "Cursor":bool=TRUE
  in  "Repair Line Col":bool
  in  "Repair Line Row":bool
  in  "Line Col":dbl=167.0
  in  "Line Row":dbl
  in  "Y-max":dbl
  in  "Y-min":dbl
  in  "X-max":dbl
  in  "X-min":dbl
  in  "Inverse":bool caption="Scan"
  in  "ViewMode":i32(ring) items=["cwViewXYPlane", "cwViewXZPlane", "cwViewYZPlane", "cwViewUserDefined"]
  in  "Plot style":i32(ring)=5 items=["cwLine"=1, "cwPoint"=2, "cwLinePoint"=3, "cwHiddenLine"=4, "cwSurface"=5, "cwSurfaceLine"=6, "cwSurfaceNormal"=7, "cwContourLine"=8, "cwSurfaceContour"=9]
  in  "ColorMapAutoScale":bool=TRUE
  in  "Max":dbl=0.6
  in  "Min":dbl=-0.8
  in  "low cutoff freq: fl":dbl=40.0 format="%0.2f"
  in  "Filter":bool caption="Scan"
  in  "Backindex":i32
  in  "Backdata":bool caption="Scan"
  in  "Odd":bool caption="Scan"
  in  "DiffX":bool caption="Scan"
  in  "DiffY":bool caption="Scan"
  in  "Abs":bool caption="Scan"
  in  "Trim data":bool caption="Scan"
  in  "Return":bool caption="Scan"
  out "No.data":i32=4316
  in  "Tab Control 2":T6(tab)
  out "Hall sensors signal":dbl[](graph)
  out "Feature Extraction":dbl(graph)=4.506984013542132
  out "Power spectral density":cluster{"f0":dbl, "df":dbl, "magnitude":dbl[]}[](graph)=[{"f0"=0.0, "df"=200.00000000000054, "magnitude"=[-40.853857162600626, -12.199208958799986, -15.853549791770895, -22.334148788959524, -24.74623025957817, -27.855813840278287, -29.764585047224674, -32.051018964466024, -33.678237652486146, -35.57019127785932, -37.00645144750946, -38.650550956743864, -39.94252614111705, -41.40083367734842, -42.57252010809867, -43.88658695227892, -44.96065948445587, -46.16358193574343, -47.16773423567689, -48.26393629227215, -49.18909203930276, -50.20791573816293, -51.07109106020317, -52.01558387805585, -52.82636733319605, -53.71130463115662, -54.48382341136326, -55.30671959801513, -56.035762587135565, -56.826969537963244, -57.505909736029395, -58.230769139410086, -58.87684093905391, -59.69202087718331, -60.27455721628562, -60.6760808674941, -61.36424440613286, -62.17406222026373, -62.716927057136296, -63.30602894178164, -63.87471123765094, -64.50994357552392, -65.06522386237984, -65.60802998414837, -66.11021257327772, -66.65308386583746, -67.15175740082151, -67.6853945423257, -68.15969152870872, -68.67730613646462, -69.18567114768769, -69.78738736721252, -70.26073806367828, -70.65115634344464, -71.00921069399396, -71.44279142777056, -71.90322786027511, -72.37581417427766, -72.75360527712758, -73.17130940093182, -73.58024978772994, -74.00230246101808, -74.43741685921852, -74.88342639959258, -75.28289334236378, -75.68485377732924, -76.12148759045964, -76.59348356575508, -76.87162197975941, -77.16600581405879, -77.5128126247831, -77.82594612885089, -78.1789288398841, -78.6361464418662, -78.98557461621381, -79.2323015773722, -79.45840571691238, -79.87478359884842, -80.45127863003998, -80.68976618175839, -80.72619710197105, -81.0372771898986, -81.37361936316289, -81.7232064302233, -82.14950432505597, -82.72300675516094, -82.798143072828, -82.76162388212515, -83.01451867235114, -83.26887935146459, -84.00428963784684, -84.58534419138822, -84.82801972180619, -85.12885439842913, -85.26729283007236, -85.53890895152426, -85.77156721499266, -85.73032010816378, -85.74718502563123, -86.20317719910659, -86.46079374028226, -86.68728533878766, -86.63506029144523, -84.42156189245563, -83.98822429228277, -86.74227281345338, -88.29703153262598, -88.16390451999237, -88.49109240107788, -88.92645147414028, -89.2538043703773, -89.33924368953402, -89.15205109531269, -89.04974968454786, -89.36118378403097, -89.45130594723022, -89.31956619833515, -89.86804945542254, -90.60181443804252, -90.48518204007559, -89.69269831857167, -89.31261096295668, -90.284073166333, -91.03288700654821, -91.7863715970652, -92.12932157081747, -91.97166324830522, -92.18497834625423, -92.38662692582702, -92.46828314190805, -93.17606364620802, -93.33632935116013, -93.09469307531646, -92.99289033072262, -92.53925855854858, -92.66020095390091, -93.38325402935942, -94.16400874663537, -94.27041543522812, -93.99779096410239, -94.588163364749, -95.15652013495539, -94.57142935960546, -94.41784088159393, -95.39274608766895, -95.4565461460801, -94.60297175781864, -95.17499935926624, -96.9173567839878, -97.10544409999835, -91.43983427956103, -96.99835520808001, -95.67648921025767, -95.35492617194473, -94.90053183466281, -95.2634133758385, -96.10997559925306, -96.21595858174788, -96.2062077738846, -96.08341357192725, -95.71873245799523, -95.9118144259523, -96.4658538020656, -96.50681310164786, -96.80210142963382, -97.78594802083504, -97.6363978170432, -96.81481071997334, -96.28346421219607, -98.20604706588458, -104.30314570786956, -98.47032453309397, -93.77308354038335, -94.8552505260802, -98.23577130890472, -98.10698505690411, -98.05059467885053, -98.92655244618743, -99.78452431447599, -100.07522375066165, -99.58175929823432, -99.28506498010196, -99.57800984194661, -99.0563432106981, -97.87640431139567, -97.37553488130055, -97.66701572100366, -99.026714399208, -98.77572913343315, -95.12688782830851, -94.82736948026019, -97.9806411626156, -100.21196731460583, -99.90494179326475, -99.96874559618007, -99.72307601679533, -99.9009835370336, -99.50539123382022, -99.8765175499591, -100.82032099735363, -101.20224408577128, -100.7467306962823, -98.45267923021426, -95.14828215512773, -93.48278446877248, -91.90099679733693, -103.12591299894856, -87.16075386301694, -86.78898826635557, -98.86785441863321, -101.7989275363122, -99.89909759418886, -100.30203283629062, -99.1565166171078, -98.23932318463417, -98.67160823668186, -99.43418311718064, -99.45593544315096, -99.22579688045809, -99.33477223383912, -100.89110461863666, -102.21015307235311, -101.13524825763531, -96.96845664774692, -93.55550985983037, -96.0947906241453, -100.71030350236043, -100.37084035747219, -100.86513708540292, -101.94021001084994, -102.69216262537851, -101.09972242194318, -99.27055818708291, -100.12691771607848, -101.77119199901541, -101.29647353713652, -100.6343023937683, -101.00350298537904, -101.95551682912195, -101.29287491232967, -100.57559523259118, -99.84254469211854, -97.87064475452146, -97.71924306810524, -99.82044164373748, -100.77323741034662, -100.68081854423352, -100.86765293354874, -101.49713302978093, -104.63246252613774]}, ...(2 in all)]
  in  "Add LF":bool
  in  "Save LF":bool caption="Save Process"
  in  "3D Surface":refnum<k7>(container)
  out "Record path":path=path "G:/Shared drives/ICSLab-Students/NDT/PECT/Data/Lift off 0-5mm 2905/PECT_default.tdms" caption="selected path"
  out "Feature extraction scan":dbl[](graph)
  in  "View Mode":bool caption="Scan"
  out "Hall sensors signal lf":dbl[][](graph)=[[-5.605666454299, -5.58381372212, -5.362192348206, -4.984186013454, -4.510518732263, -3.9949199935, -3.460435027485, -2.926402311829, -2.408485872231, -1.916032433375, -1.450331032401, -1.010769125855, -0.597314353399, -0.214317745761, 0.140541386678, 0.46484580976, 0.769296129854, 1.044803345105, 1.29668552516, 1.53087311312, 1.745109973007, 1.938687033337, 2.118823951247, 2.283651349667, 2.440517808795, 2.578819449105, 2.699458721829, 2.811524662039, 2.92014194018, 3.013707520222, 3.099892293085, 3.177116953863, 3.254825084521, 3.323734252653, 3.386390678548, 3.441762978617, 3.49436344594, 3.541903701271, 3.583674668258, 3.62099780372, 3.660029168596, 3.694741623694, 3.726231011788, 3.755013023409, 3.781667810677, 3.807935831095, 3.829788246702, 3.844711062007, 3.864726329201, 3.882775524237, 3.898504109069, 3.913072388959, 3.92899435914, 3.94755924813, 3.959645764797, 3.965801830667, 3.974181815878, 3.987106331937, 3.993810320369, 4.000675462538, 4.005961299813, 4.017338742318, 4.025750959244, 4.031971487558, 4.038772168915, 4.042478701457, 4.048280230673, 4.05121322605, 4.052985915579, 4.059625443652, 4.06581374175, 4.068811198685, 4.072646654355, 4.077320108797, 4.082444793433, 4.083218330733, 4.082928254186, 4.08605463411, 4.090051243565, 4.091243780255, 4.093113162163, 4.096723003067, 4.10484514507, 4.105715374565, 4.104619529898, 4.103201378093, 4.107745910102, 4.108777293189, 4.109518599804, 4.10729467995, 4.115674667933, 4.117028358294, 4.116770512461, 4.118382048665, 4.120283661357, 4.119800200491, 4.120638199331, 4.119767969788, 4.123087734329, 4.125311654297, 4.126762036878, 4.125247192836, 4.128760341783, 4.130500800946, 4.128341342423, 4.126278576011, 4.127728958591, 4.130017340027, 4.13204787569, 4.130984261808, 4.133530489102, 4.140685710148, 4.138365097867, 4.135593255405, 4.134819718021, 4.134594103027, 4.136270100697, 4.137237022458, 4.132628028851, 4.140395633556, 4.14158817036, 4.139976634038, 4.140717940722, 4.140975786579, 4.140621248543, 4.137881636932, 4.139912172614, 4.142071631184, 4.144198859098, 4.143876551839, 4.142426169197, 4.145326934482, 4.145907087585, 4.143554244597, 4.141588170308, 4.14191047754, 4.144295551238, 4.14632608698, 4.145294703774, 4.146487240651, 4.154544922318, 4.150580542897, 4.146326086949, 4.145649241749, 4.147647546823, 4.145939318333, 4.147325239555, 4.144069936296, 4.150193774197, 4.150097081997, 4.149613621037, 4.148388853426, 4.149484698165, 4.148807852881, 4.146551702092, 4.14761531608, 4.151902002577, 4.152997847295, 4.153030078003, 4.150419389178, 4.15367469255, 4.153384616012, 4.149516928845, 4.148259930546, 4.150967311518, 4.15180531039, 4.153642461779, 4.152482155641, 4.152707770772, 4.158058071445, 4.156156458543, 4.15286892434, 4.151321849516, 4.152707770794, 4.152804462995, 4.151966464091, 4.151740849026, 4.156027535645, 4.156253150722, 4.153900307617, 4.153287923787, 4.154125922699, 4.153449077442, 4.151354080272, 4.153030078083, 4.156317612101, 4.157316764638, 4.157413456793, 4.155415151752, 4.156672150126, 4.157252303177, 4.153932538314, 4.151998694777, 4.15435153779, 4.156704380794, 4.156736611522, 4.157123380238, 4.157316764613, 4.161571220631, 4.158348147899, 4.156253150616, 4.155382921013, 4.1567688423, 4.156478765785, 4.156897765193, 4.155060613787, 4.15957291561, 4.158799378121, 4.157348995341, 4.156446534968, 4.157606841156, 4.155995304819, 4.153835846177, 4.155350690368, 4.160120837839, 4.160056376399, 4.159927453471, 4.157961379157, 4.160185299336, 4.158122532786, 4.156929995881, 4.15483499869, 4.156833303714, 4.157671302607, 4.158863839484, 4.157929148393, 4.160056376384, 4.162022450817, 4.160281991487, 4.157510148982, 4.156349842808, 4.157510149001, 4.157542379743, 4.157348995344, 4.157961379158, 4.160443145215, 4.160572068084, 4.159862992045, 4.159637376915, 4.159476223281, 4.158863839497, 4.156414304278, 4.157896917743, 4.161184451811, 4.161990220002, 4.160281991445, 4.159540684784, 4.161603451331, 4.160604298745, 4.158348147871, 4.14593931828, 4.124505886212, 3.902532947463, 3.526110666805, 3.058701513854, 2.542237680027, 2.008788622196, 1.473502631793, 0.955524568977, 0.45901206943, -0.008396297786, -0.448666655325, -0.859768503244, -1.240412621149, -1.59369314171, -1.921286040481, -2.2225144437, -2.497765083525, -2.751743614071, -2.986673927337, -3.201589066875, -3.397391462407, -3.573823234133, -3.737942916417, -3.889267026352, -4.027731082679, -4.150530973424, -4.266433499351, -4.373085790051, -4.47035890998, -4.557156993943, -4.637347752427, -4.711027871951, -4.778455194505, -4.838952862737, -4.895034893163, -4.948248373645, -4.995821430036, -5.039526767653, -5.079751157428, -5.117687147494, -5.151433102162, -5.181891489982, -5.210512709547, -5.236716599839, -5.262469257845, -5.281936851307, -5.301211060077, -5.322000133444, -5.342176817567, -5.357744452311, -5.370991446749, -5.384109517601, -5.398516834667, -5.412053912328, -5.42140094248, -5.432069450042, -5.441867717064, -5.451956064977, -5.460046082532, -5.467491477305, -5.476774047997, -5.481866569342, -5.487700407543, -5.491825994796, -5.499110235107, -5.504138295006, -5.507361410262, -5.513163018152, -5.518255540568, -5.524057148756, -5.527763731684, -5.530084375053, -5.534919048777, -5.537723159497, -5.539238023941, -5.539463642082, -5.543556999286, -5.547940437053, -5.550937935023, -5.551840407528, -5.555224679491, -5.557674247779, -5.560349434504, -5.559446961945, -5.562315535415, -5.563024620799, -5.566344430613, -5.567440290292, -5.570244401573, -5.572113809136, -5.573274130898, -5.573241899744, -5.573403055571, -5.57475676451, -5.578237730445, -5.575594774773, -5.578656735549, -5.579526976975, -5.584264958634, -5.583072405266, -5.584555038969, -5.584941812928, -5.586875682928, -5.58471619476, -5.583652566322, -5.585650898565, -5.588487241255, -5.591452508778, -5.59013103086, -5.590388880186, -5.59367645934, -5.593708690668, -5.591097966217, -5.591226890753, -5.592612830807, -5.594063233318, -5.594127695792, -5.59722188804, -5.598446672442, -5.598607828121, -5.596480570971, -5.595126861875, -5.596802882649, -5.598511134706, -5.596190490454, -5.598317747618, -5.600316080065, -5.601573095846, -5.602668955499, -5.600606160639, -5.600187155372, -5.603087960653, -5.600348311286, -5.596802882761, -5.601186321636, -5.602314412561, -5.605376373778, -5.6029268048, -5.602959035997, -5.604635056809, -5.605698685577, -5.602346644163, -5.602765649149, -5.605408605021, -5.606601158184, -5.60505406216, -5.60776148048, -5.609050727289, -5.607761480371, -5.605150755611, -5.603249116567, -5.606343308829, -5.609566425999, -5.60353919708, -5.60847056607, -5.609340807675, -5.61124244698, -5.609211883037, -5.60792263619, -5.607278012748, -5.609888737585, -5.607987098557, -5.606407771265, -5.608116023225, -5.611016828589, -5.611725914407, -5.608921802479, -5.60908295835, -5.610887903906, -5.610662285818, -5.609308576813, -5.60847056628, -5.611725914421, -5.612080457216, -5.610243280578, -5.613820940653, -5.614239945882, -5.611339140433, -5.609115189613, -5.607245781702, -5.610501129841, -5.613788709408, -5.609340807733, -5.611919301392, -5.613530859955, -5.61565811745, -5.612402769031, -5.610565592197, -5.611693683171, -5.612660618329, -5.611758145538, -5.61063005455, -5.613144085926, -5.614304408075, -5.615271343246, -5.611596989671, -5.613240779413, -5.613401935285, -5.613788709387, -5.613015161416, -5.612886236743, -5.61482010689, -5.617656449971, -5.613305241831, -5.616334972052, -5.616818439683, -5.614755644605, -5.610339974209, -5.610146587069, -5.614433332772, -5.616463896697, -5.612112688479, -5.614981262697, -5.615948197886, -5.619880401116, -5.614046558826, -5.612370537823, -5.612628387144, -5.614981262677, -5.614787875726, -5.616367203107, -5.615464730318, -5.61804322403, -5.61723744472, -5.611629220854, -5.613627553505, -5.615013493844, -5.614014327587, -5.613627553752, -5.614755644654, -5.617624218884, -5.618687847465, -5.616786208383, -5.616334971936, -5.617559756569, -5.615432499247, -5.610372205464, -5.611306909303, -5.61665728361, -5.616979595419, -5.614691182253, -5.617044057748, -5.61768868125, -5.620363868727, -5.615271343393, -5.611242446924, -5.616012660198, -5.616753977156, -5.615206880995], [-5.602024332038, -5.575240232006, -5.349589976818, -4.975000158759, -4.509165030327, -3.989634121078, -3.454375625029, -2.917152070333, -2.403393412496, -1.911197825708, -1.440371750737, -0.998231399396, -0.586452627799, -0.211868218223, 0.14276529916, 0.471356392899, 0.77119773562, 1.049637935862, 1.298812745142, 1.531517725275, 1.747333885159, 1.945391001223, 2.121885860059, 2.280621671002, 2.431009773202, 2.570020485962, 2.694269588955, 2.810461050813, 2.909634748729, 3.00835723177, 3.09734607115, 3.181242478576, 3.252117708573, 3.314612973168, 3.379235469103, 3.437379606677, 3.491946144969, 3.535876563608, 3.578582219945, 3.620192036543, 3.657869712368, 3.696127543557, 3.71972041146, 3.747632193836, 3.776317514665, 3.801586383029, 3.82424456592, 3.840521070644, 3.859633877883, 3.879101223737, 3.89544219189, 3.91246000547, 3.919002839308, 3.931927353602, 3.946946864517, 3.958227613387, 3.969218286176, 3.975084275893, 3.985784872615, 3.996485469666, 4.006734836952, 4.013406594982, 4.01508259222, 4.023269194111, 4.031262411879, 4.040706012002, 4.040706011974, 4.04673315622, 4.053050377024, 4.058142830622, 4.065136896654, 4.06391212935, 4.064717897282, 4.069488043799, 4.0758697264, 4.080188642941, 4.07683664805, 4.080478719398, 4.084507559508, 4.087408324423, 4.090728088719, 4.089213244833, 4.088923168311, 4.092984239217, 4.096690772228, 4.099398152881, 4.09652961865, 4.100365074556, 4.105489759463, 4.10909960036, 4.109035138905, 4.107778140751, 4.109292984769, 4.111935904079, 4.118607663765, 4.116029205937, 4.11444990044, 4.118510971587, 4.120767122244, 4.124344732573, 4.1179630493, 4.120380353507, 4.119510123974, 4.124312501841, 4.126697575437, 4.12141173674, 4.122056351162, 4.123957963872, 4.126181883837, 4.129082649039, 4.122378658418, 4.124119117489, 4.125537269352, 4.12927603338, 4.130565262354, 4.127696727924, 4.127664497223, 4.131757799239, 4.13604448561, 4.135238717441, 4.131338799811, 4.134787487358, 4.13356271985, 4.139783249704, 4.13768825266, 4.136334562134, 4.135689947643, 4.139525403959, 4.141684862491, 4.136141177805, 4.136656869339, 4.136753561528, 4.139041943011, 4.142297246284, 4.136946945923, 4.138365097786, 4.137301483853, 4.140750171448, 4.142619553549, 4.137204791713, 4.136592407895, 4.138880789426, 4.142297246274, 4.143135245138, 4.140750171493, 4.14065347933, 4.140750171545, 4.147486393141, 4.146003779738, 4.142522861414, 4.14249063066, 4.145842626181, 4.150193774132, 4.147744239007, 4.147421931715, 4.144037705495, 4.146777317204, 4.150870619342, 4.144392243473, 4.14600377973, 4.141620401077, 4.148163238351, 4.148969006492, 4.146648394271, 4.146132702635, 4.143457552404, 4.14597154899, 4.147002932228, 4.145391395947, 4.143264168055, 4.14377985969, 4.14977477465, 4.149388005942, 4.14800208478, 4.146164933364, 4.147679777582, 4.150580542838, 4.151289618795, 4.149033467988, 4.147293008785, 4.149742543973, 4.155382921038, 4.151998694841, 4.151450772455, 4.14729300879, 4.151257388089, 4.151225157316, 4.149130160135, 4.149839236101, 4.146197164106, 4.150645004244, 4.152417694193, 4.150419389172, 4.149194621601, 4.147873161825, 4.150322696996, 4.149194621575, 4.150322696999, 4.146455009892, 4.14864669927, 4.151998694768, 4.153706923273, 4.152030925518, 4.149033467977, 4.150709465782, 4.152611078584, 4.153126770163, 4.152514386384, 4.150097081938, 4.153803615447, 4.155253998112, 4.15567299762, 4.15344907746, 4.150097081933, 4.152192079119, 4.153126770154, 4.150580542796, 4.151644156762, 4.148259930549, 4.152127617645, 4.152901155072, 4.15464161431, 4.149807005379, 4.148646699229, 4.152933385815, 4.15041938915, 4.152385463467, 4.149291313765, 4.150677234991, 4.153545769644, 4.154190384159, 4.156607688636, 4.150709465719, 4.153352385301, 4.153900307632, 4.155963074077, 4.153964769061, 4.152288771327, 4.155092844492, 4.156607688623, 4.156639919416, 4.156156458475, 4.151998694758, 4.152997847262, 4.153771384682, 4.15406146122, 4.151676387492, 4.149710313214, 4.153320154526, 4.15351353887, 4.143812090355, 4.120477045693, 3.893411657331, 3.520276913394, 3.051352924434, 2.535759322851, 1.99544514708, 1.46451029241, 0.949465215198, 0.455789008451, -0.010878055496, -0.452695484582, -0.862862645848, -1.242926613616, -1.594369986227, -1.922091808358, -2.225705287226, -2.499570006483, -2.751646921727, -2.983192999539, -3.198140367456, -3.3959088429, -3.575209161899, -3.737394991121, -3.886205089289, -4.025797226592, -4.154237532754, -4.265434339323, -4.369346996246, -4.464267252145, -4.552999194094, -4.633963495538, -4.706160986656, -4.773104842185, -4.833409122577, -4.892682026148, -4.946056661378, -4.989729757629, -5.031114456416, -5.071048764713, -5.109564912831, -5.142698475301, -5.17338247958, -5.20126238243, -5.227853044833, -5.253895781824, -5.278617046398, -5.294313600548, -5.313168805936, -5.332024013049, -5.351556075634, -5.366414626189, -5.378823611772, -5.392811923752, -5.403867203361, -5.418919144717, -5.428169481807, -5.434035549461, -5.443253656151, -5.450860206061, -5.463752664227, -5.466041075696, -5.473164159232, -5.480577323405, -5.485476458206, -5.494501180478, -5.496886285711, -5.499754858259, -5.502333350372, -5.508425038357, -5.515870435044, -5.516096053176, -5.520479490293, -5.523638143668, -5.529181902642, -5.534371119053, -5.53372649586, -5.536079370429, -5.538432245002, -5.543492536993, -5.549358608157, -5.546361110222, -5.550776779213, -5.551260246652, -5.556449463714, -5.557384167375, -5.556578388334, -5.557287473829, -5.55851225802, -5.564410560797, -5.564378329644, -5.563346932427, -5.565441958059, -5.566441124171, -5.570760100192, -5.569503084836, -5.570856793675, -5.567311365578, -5.571404723377, -5.574692302197, -5.573918754246, -5.573564211381, -5.57398321668, -5.577431951374, -5.580751761373, -5.578334423858, -5.579784826335, -5.579784826309, -5.58262116897, -5.586005441467, -5.584748425918, -5.583523641598, -5.584264958436, -5.587681462196, -5.587488075144, -5.58613436612, -5.587745924446, -5.585199662264, -5.590969041205, -5.590872347718, -5.589002940054, -5.585973210322, -5.587810386858, -5.590936810101, -5.590388880299, -5.589969875089, -5.589131864696, -5.591033503516, -5.59316076063, -5.592580599612, -5.592741755417, -5.589744256936, -5.59454670098, -5.596512802204, -5.595030168347, -5.594514469694, -5.595997103419, -5.598640059276, -5.600445004756, -5.59760866189, -5.597640893071, -5.594514469736, -5.59996153725, -5.600896241129, -5.597866511247, -5.597866511243, -5.597157425539, -5.6000259996, -5.601025165868, -5.597769817832, -5.596061565893, -5.59612602819, -5.599187989268, -5.600187155458, -5.598640059336, -5.596641726853, -5.599993768402, -5.601444171047, -5.601121859301, -5.599091295634, -5.598672290595, -5.599220220449, -5.60366812178, -5.603764815205, -5.602797880123, -5.603313578862, -5.605376373765, -5.606214384155, -5.604570594521, -5.603442503627, -5.60260449318, -5.604022664612, -5.606859007573, -5.601476402205, -5.603442503535, -5.601637558036, -5.605150755605, -5.605666454344, -5.602604493217, -5.60108962827, -5.601927638676, -5.604216051724, -5.605182986775, -5.602411106132, -5.60092847238, -5.60334581003, -5.607213550546, -5.606536695862, -5.604925137326, -5.604054895874, -5.605376373837, -5.606955701104, -5.608696184281, -5.607406937447, -5.606149921842, -5.608309410319, -5.611596989693, -5.607761480386, -5.607890405163, -5.605247449114, -5.607568093354, -5.609147420745, -5.606955701135, -5.606085459545, -5.602991267174, -5.607568093456, -5.610082124741, -5.605408604974, -5.604667288182, -5.60341027254, -5.60769701809, -5.607116856958, -5.604957368563, -5.604699519264, -5.605827610141, -5.610436667559, -5.611210215651, -5.606568927044, -5.605730916642, -5.607600324506, -5.611725914434, -5.609566425916, -5.609888737596, -5.606955701072, -5.608663953144, -5.613144085957, -5.611725914447, -5.608792877967, -5.605763147886, -5.607471399816, -5.611500296238, -5.606633389434, -5.607825942858, -5.603087960778, -5.607600324633, -5.609727581858, -5.607535862228, -5.606665620765, -5.603700353068, -5.609534194806, -5.610662285706, -5.606182153084, -5.606955701183, -5.607858173921, -5.610565592351, -5.612950698892, -5.610630054556, -5.607535862125, -5.608954033682, -5.612563924893], [-5.589002940076, -5.565280802314, -5.328156278181, -4.941931085254, -4.460173916087, -3.930941605187, -3.384402426938, -2.841474145742, -2.317401760689, -1.815956066037, -1.346193698632, -0.900314664801, -0.488729334476, -0.103541090928, 0.247353643671, 0.574462110353, 0.874238982334, 1.150004040044, 1.401725070403, 1.630659076875, 1.842317498257, 2.033348352108, 2.212292750612, 2.37251118377, 2.519063855337, 2.65330444809, 2.775039574115, 2.887879061417, 2.986794925222, 3.080263822841, 3.162033004314, 3.242545200886, 3.311937827603, 3.377720627447, 3.435058997869, 3.490076765507, 3.538906247755, 3.582965593169, 3.623705181544, 3.659545708239, 3.696611003946, 3.726843395033, 3.757623709934, 3.783085961435, 3.807903600318, 3.83204439582, 3.852285277355, 3.872139391377, 3.885805210592, 3.903403176577, 3.915715306999, 3.934505810379, 3.944755176239, 3.956551616412, 3.966962136324, 3.978178424282, 3.988202176125, 3.996098701083, 4.004446456138, 4.008668679852, 4.017338742327, 4.023398116967, 4.031133488947, 4.035678020046, 4.040609319827, 4.047023232663, 4.049053767938, 4.054436297933, 4.05659575608, 4.06362205287, 4.064814589504, 4.069326890286, 4.071744194223, 4.075740803515, 4.080027489342, 4.082573716269, 4.08328279212, 4.083186099963, 4.086344710629, 4.087053786481, 4.092049548293, 4.093209854341, 4.094789159643, 4.095627158421, 4.097689924611, 4.103072455215, 4.10178322633, 4.104619529883, 4.10084853539, 4.10510299075, 4.105070760052, 4.108519447331, 4.109776445557, 4.111130135912, 4.110775597941, 4.111806981095, 4.112677210636, 4.111742519644, 4.116061436583, 4.114739977, 4.11631928241, 4.116383743829, 4.117737434192, 4.122056351202, 4.120348122806, 4.121476198127, 4.117060589005, 4.120863814383, 4.119767969762, 4.12370011809, 4.122604273576, 4.123603425922, 4.122572042736, 4.125472807927, 4.127922342969, 4.126052960963, 4.127696727866, 4.123474503022, 4.127632266445, 4.127438882118, 4.128212419465, 4.130533031668, 4.129630571372, 4.131016492499, 4.1296950328, 4.131757799182, 4.128663649612, 4.133272643251, 4.130436339533, 4.132853643884, 4.130694185279, 4.133530489038, 4.136334562132, 4.134271795716, 4.135561024693, 4.131403261198, 4.133756104096, 4.134175103503, 4.135689947578, 4.135883332055, 4.135689947623, 4.134626333651, 4.136914715165, 4.140621248577, 4.137849406195, 4.13923532734, 4.133272643241, 4.138332867053, 4.136495715747, 4.138558482116, 4.137623791159, 4.13820394421, 4.138945250825, 4.138429559239, 4.139622096071, 4.137430406761, 4.139203096642, 4.13823617495, 4.140750171521, 4.137913867672, 4.139267558069, 4.143264168074, 4.140460094963, 4.141330324498, 4.136302331379, 4.139622096064, 4.138880789361, 4.141717093196, 4.141684862597, 4.140524556392, 4.139138635168, 4.141620401051, 4.143844321132, 4.142651784266, 4.143296398731, 4.13871963577, 4.142684014973, 4.140943555821, 4.142490630615, 4.143103014489, 4.140331172035, 4.143973244, 4.141652631766, 4.14316747588, 4.141491478132, 4.144553397053, 4.142103861989, 4.14458562783, 4.142587322834, 4.143522013822, 4.145262473076, 4.144231089868, 4.145326934469, 4.14033117203, 4.143296398755, 4.142780707149, 4.144617858491, 4.144746781509, 4.143844321132, 4.143070783669, 4.142748476419, 4.146455009927, 4.146229394837, 4.145971548974, 4.141008017262, 4.147067393656, 4.144263320519, 4.14622939478, 4.14542362677, 4.143715398218, 4.14394101327, 4.143715398184, 4.14481124288, 4.144005474725, 4.145455857398, 4.144843473672, 4.14548808814, 4.144488935629, 4.145036857929, 4.1475186239, 4.144843473641, 4.146422779156, 4.141330324528, 4.145617011016, 4.143296398754, 4.147679777445, 4.14719631671, 4.144940165838, 4.144650089246, 4.145874856826, 4.14719631665, 4.14722854738, 4.146938470763, 4.142329477012, 4.146068241145, 4.146616163492, 4.147518623819, 4.146551702164, 4.144392243476, 4.146358317694, 4.143360860218, 4.146261625501, 4.145455857361, 4.148066546159, 4.145939318326, 4.148582237804, 4.14690624004, 4.148614468493, 4.149549159616, 4.147486393143, 4.135754409054, 4.10561868235, 3.879584684347, 3.489980073445, 3.010710069456, 2.482578780776, 1.932692139007, 1.390508819361, 0.865762333086, 0.367058137851, -0.107859994347, -0.55028985094, -0.967161044838, -1.345097855537, -1.698604064809, -2.021910354857, -2.324170218454, -2.601354781489, -2.852948310338, -3.08465561587, -3.292770116631, -3.487057723343, -3.660911081343, -3.822613499235, -3.969554252763, -4.102216783327, -4.223566318254, -4.334924312073, -4.438772537922, -4.5301151811, -4.620555392738, -4.693300806808, -4.765304931116, -4.826286061324, -4.88610689105, -4.941318695039, -4.991534697546, -5.035143341095, -5.074400797622, -5.112433479973, -5.149015769906, -5.184631133656, -5.20890115416, -5.234653808739, -5.257408973034, -5.281679002716, -5.30446640334, -5.322000133465, -5.342853671289, -5.354424646068, -5.373924479721, -5.385656611967, -5.397356514006, -5.407606015236, -5.419434842904, -5.427814939226, -5.437613206328, -5.448185021198, -5.454856868114, -5.46610553804, -5.470037737853, -5.477547595411, -5.481318639876, -5.487023553554, -5.493727632804, -5.497595371034, -5.503300285053, -5.505105229637, -5.510810143875, -5.514387801963, -5.521800967783, -5.520447259179, -5.524411691352, -5.523380294417, -5.531083541222, -5.533533109038, -5.534048807405, -5.540462807998, -5.538303320361, -5.543073531928, -5.543782617461, -5.545974336455, -5.546264416798, -5.547682587851, -5.549874306706, -5.550164387277, -5.553677583856, -5.553903201966, -5.561187444639, -5.557964328249, -5.561896530132, -5.559027956662, -5.560768439521, -5.562057685953, -5.564442792109, -5.565667576229, -5.562927927385, -5.564797335, -5.567698139692, -5.571694803945, -5.569825396313, -5.570598944329, -5.567633677268, -5.571082411953, -5.57385429201, -5.572951819284, -5.576465016297, -5.573048512779, -5.577625338243, -5.574885689174, -5.578044343555, -5.575884855312, -5.577238564254, -5.576626172107, -5.576336091691, -5.579365821304, -5.57849557973, -5.583942646831, -5.581267459985, -5.58300794295, -5.58017160035, -5.580912917321, -5.58394264687, -5.583136867813, -5.584393883156, -5.580945148378, -5.583136867785, -5.583265792435, -5.588551703732, -5.585489742773, -5.584619501378, -5.583040174158, -5.585489742997, -5.58735915062, -5.587520306354, -5.588068236187, -5.58494181297, -5.589196327074, -5.587359150512, -5.589647563547, -5.58900294007, -5.586392215469, -5.5881326985, -5.586037672732, -5.589969875155, -5.588712859532, -5.592967373724, -5.58945417634, -5.592838448999, -5.589454176353, -5.590550036236, -5.592741755541, -5.591033503682, -5.592902911361, -5.589583101071, -5.590550036246, -5.591259121877, -5.595481404863, -5.592902911307, -5.590969041355, -5.590743423073, -5.59299960497, -5.595223555633, -5.592129363404, -5.595384711309, -5.590840116563, -5.594965706227, -5.593257454208, -5.594836781541, -5.593966539922, -5.592935142482, -5.593160760655, -5.592226056874, -5.594578932129, -5.593289685342, -5.596577264566, -5.594159926883, -5.595868178802, -5.594353313858, -5.593934308844, -5.597189656721, -5.595191324311, -5.598221054126, -5.592806217831, -5.595578098334, -5.595094630797, -5.597995435953, -5.595997103432, -5.596190490523, -5.593805384007, -5.595868178914, -5.599123526915, -5.596802882777, -5.598962371001, -5.595094630744, -5.59760866197, -5.596706189233, -5.597963204907, -5.597898742487, -5.596126028159, -5.597608661912, -5.595513636078, -5.59867229056, -5.596061565861, -5.600219386654, -5.596802882712, -5.599703687927, -5.597221887886, -5.597092963247, -5.599316913845, -5.598478903504, -5.600348311297, -5.59583594767, -5.597576430782, -5.597286350263, -5.598833446348, -5.598736752789, -5.596512802171, -5.596093796991, -5.596738420393, -5.60083177889, -5.598833446376, -5.599606994436, -5.596738420368, -5.598930139892, -5.598188822989, -5.59999376846, -5.599316913889, -5.599413607358, -5.599284682683, -5.59860782823, -5.601476402242, -5.597834280141, -5.600541698314, -5.598994602241, -5.600670623036, -5.599155758005, -5.598672290523, -5.599864843721, -5.599735919095, -5.603023498345, -5.598414441139, -5.600735085323, -5.599026833323, -5.600831778866, -5.599542532014, -5.598382209951, -5.598059898276, -5.598382209953, -5.6013152464]]
  in  "Open":bool
  in  "Filter lf":bool=TRUE caption="Scan"
  in  "Low cutoff freq: fl":dbl=40.0
  in  "Tab Control":T7(tab)
  out "Start Pos X":dbl
  out "Start Pos Y":dbl
  in  "Step X":dbl=1.0
  in  "Y - length":dbl=20.0
  in  "X - length":dbl=20.0
  in  "Step Y":dbl=1.0
  in  "Multiplier":dbl=10.0
  out "Cur. Pos Y":dbl format="%#_4g"
  in  "Speed (mm/s)":dbl=3.0
  in  "Travel per Pulse (mm)":dbl=0.004
  in  "COM Y":refnum<visa-resource-name>="COM3"
  in  "COM X":refnum<visa-resource-name>="COM4"
  out "Completed":bool
  out "No. X":i32=7
  out "No. Y":i32=2
  in  "Baud Rate":u32=9600
  out "Cur. Pos X":dbl format="%#_4g"
  in  "DAQ Pulser":bool=TRUE
  in  "No. Samples":dbl=500.0
  out "Sample per Channel AO":dbl=40000.0
  in  "Pulser Cycles":i32=10
  out "Actual Sample Rate":dbl=100000.0 format="%0.2f"
  in  "Physical Channel":tag="Dev3/ai1:2"
  in  "Min Voltage":dbl=-10.0
  in  "Max Voltage":dbl=10.0
  in  "Terminal Configuration":i32(ring)=10083 items=["default"=-1, "RSE"=10083, "NRSE"=10078, "Differential"=10106, "Pseudodifferential"=12529]
  in  "Sample Clock Source 2":tag="OnboardClock"
  in  "Sample Rate":dbl=100000.0
  out "Actual Sample Rate 2":dbl=800000.0 format="%0.2f"
  in  "Physical Channel(s)":tag="Dev3/ao0:1"
  in  "Min Voltage 2":dbl=-10.0
  in  "Max Voltage 2":dbl=10.0
  in  "Sample Clock Source":tag="OnboardClock"
  in  "Sample Rate 2":dbl=800000.0 format="%#_6p"
  # "Pulse Shape"
  # "Trigger Settings"
  # "Data Processing"
  # "Time gate = %T/2"
  # "3D Surface"
  # "Process"
  # "Repair line"
  # "Hall Sensors Signal"
  # "Feature Extraction"
  # "Power Spectal Density"
  # "COM Setting"
  # "Speed Setting"
  # "Scan Setting"
  # "Pulser Channel"
  # "Pulser Timming"
  # "Sensor Channel"
  # "DAQ Timming"
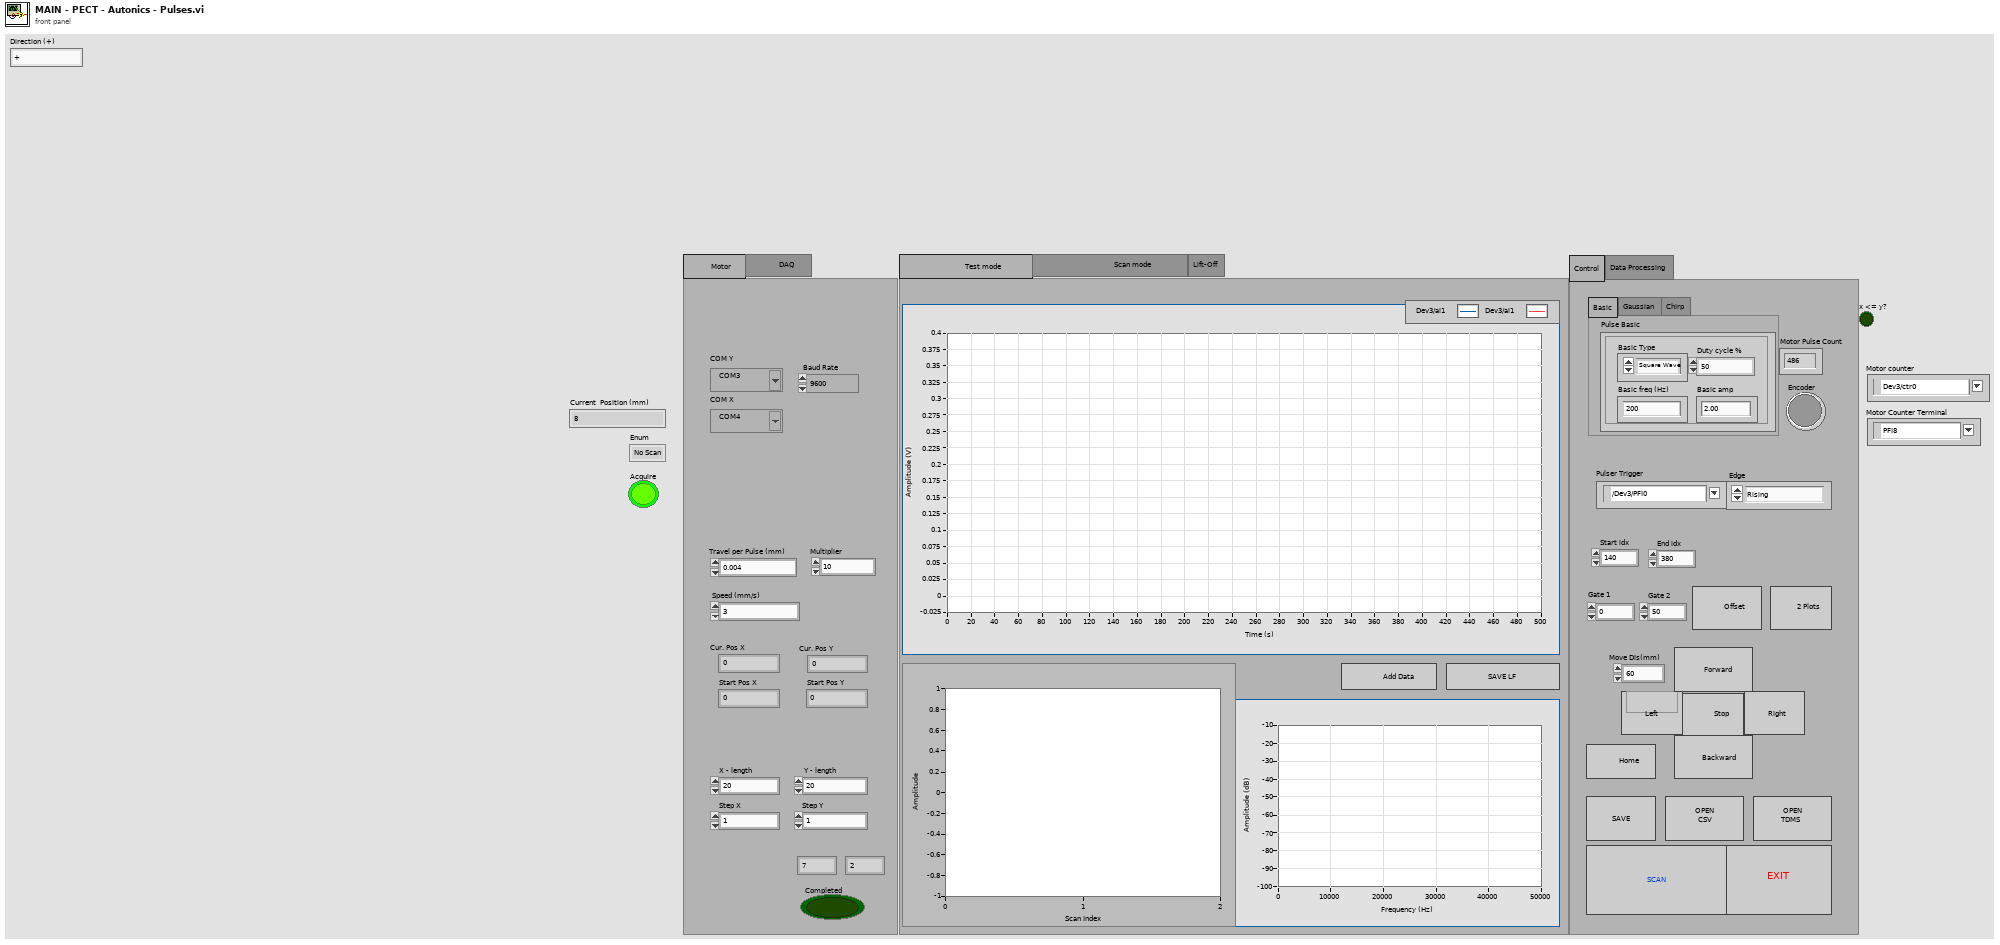
[diagram p1: front panel]
types:
  T1 = enum16{"No Scan", "Move X", "Wait X", "Move Y", "Wait Y"}
  T2 = typedef "Control 1.ctl" = dbl
  T3 = cluster{"Basic amp":T2, "Duty cycle %":dbl, "Basic freq (Hz)":u16, "Basic Type":u16}
  T4 = cluster{"Gauss amp":dbl, "Gauss Nor. Band":dbl, "Gauss atten (dB)":dbl, "Gauss freq (Hz)":dbl}
  T5 = cluster{"Chirp amp":dbl, "Chirp f2":dbl, "Chirp f1":dbl}
  T6 = enum32{"                    Test mode                   ", "                          Scan mode                      ", "Lift-Off"}
  T7 = enum32{"        Motor      ", "          DAQ        "}
  T8 = enum16{"open", "open or create", "create or replace", "create", "open (read-only)"}
  T9 = cluster{"averaging mode":u16, "weighting mode":u16, "number of averages":u32}
  T10 = cluster{"dB On (F)":bool, "unwrap phase (F)":bool, "convert to degree (F)":bool}
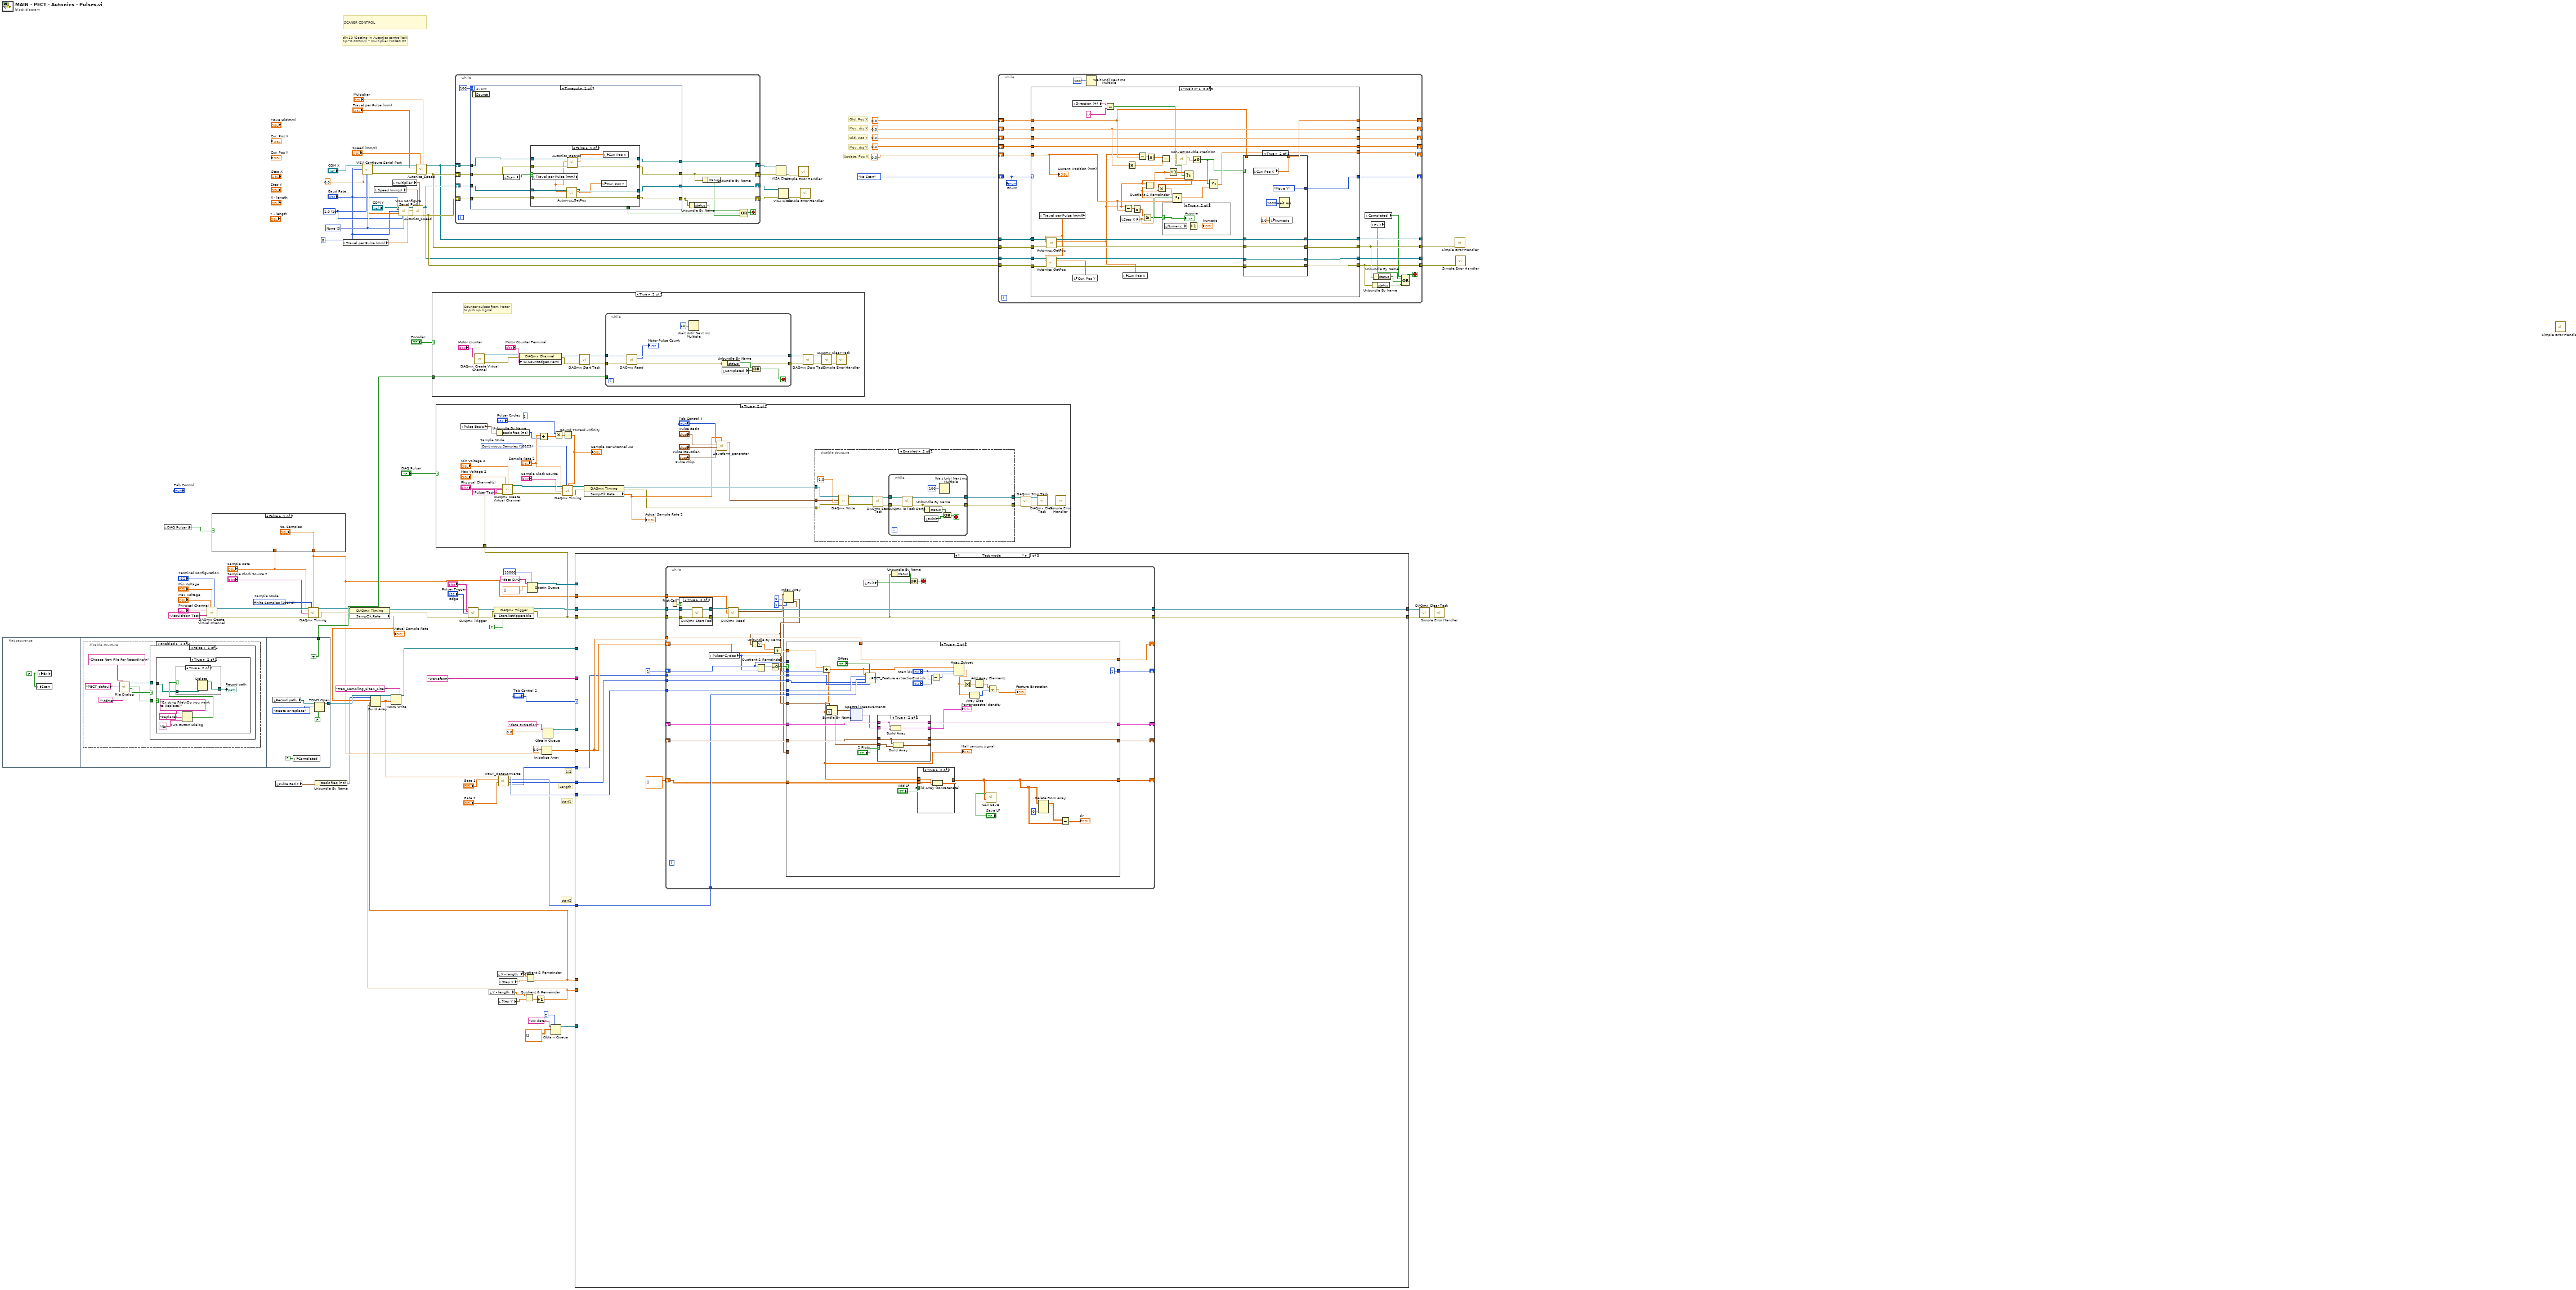
[diagram p0: block diagram]
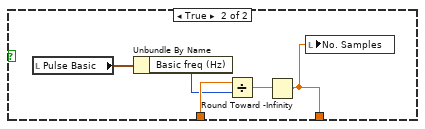
[diagram p3: hidden frame]
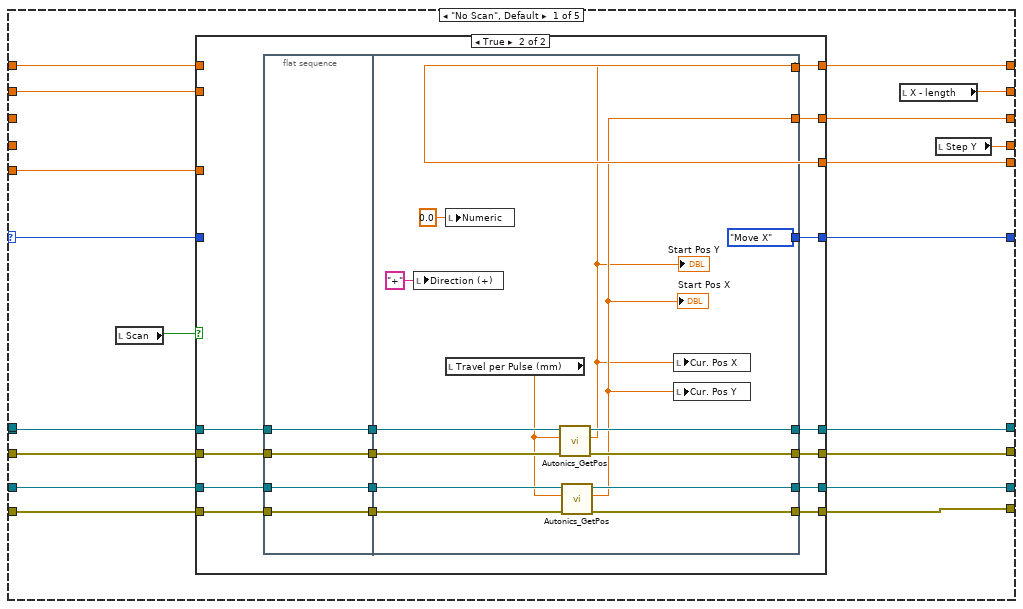
[diagram p4: hidden frame]
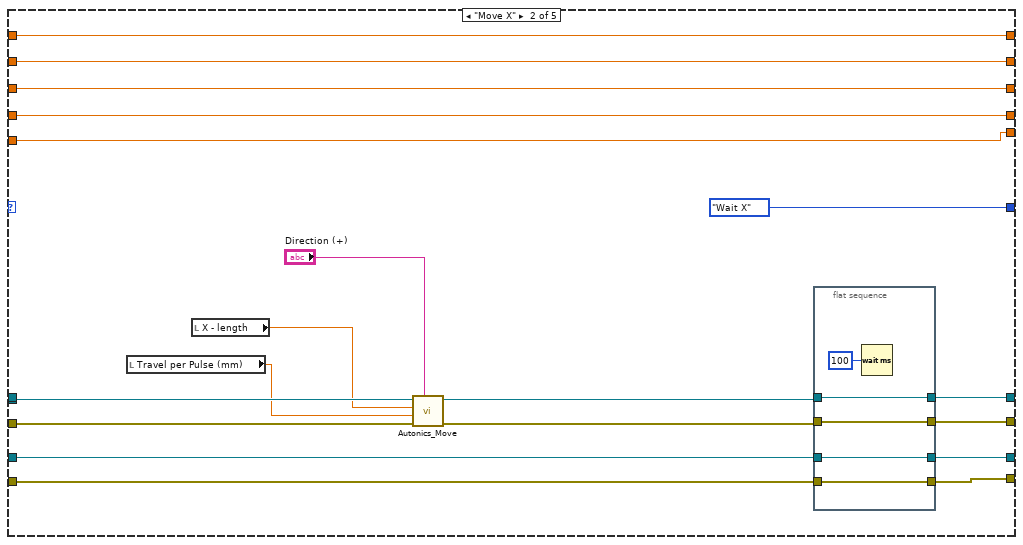
[diagram p6: hidden frame]
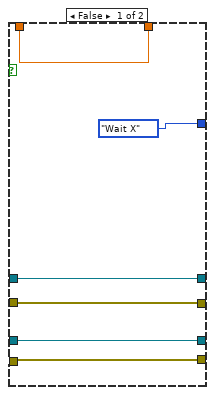
[diagram p8: hidden frame]
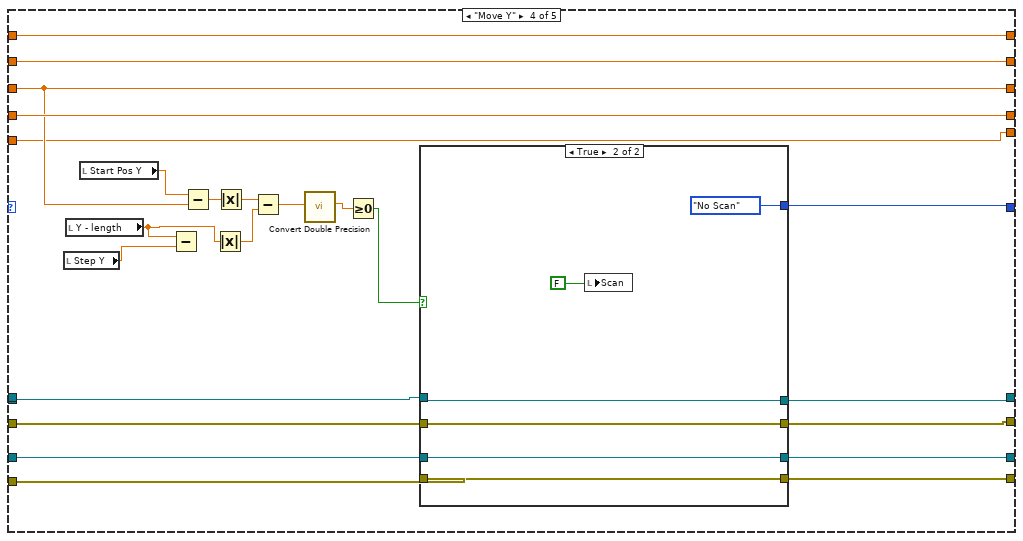
[diagram p9: hidden frame]
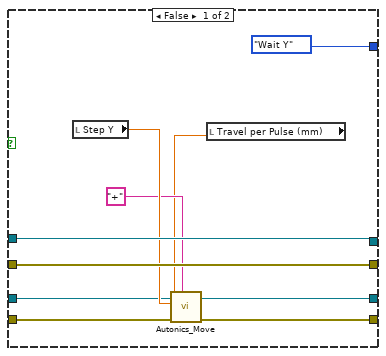
[diagram p10: hidden frame]
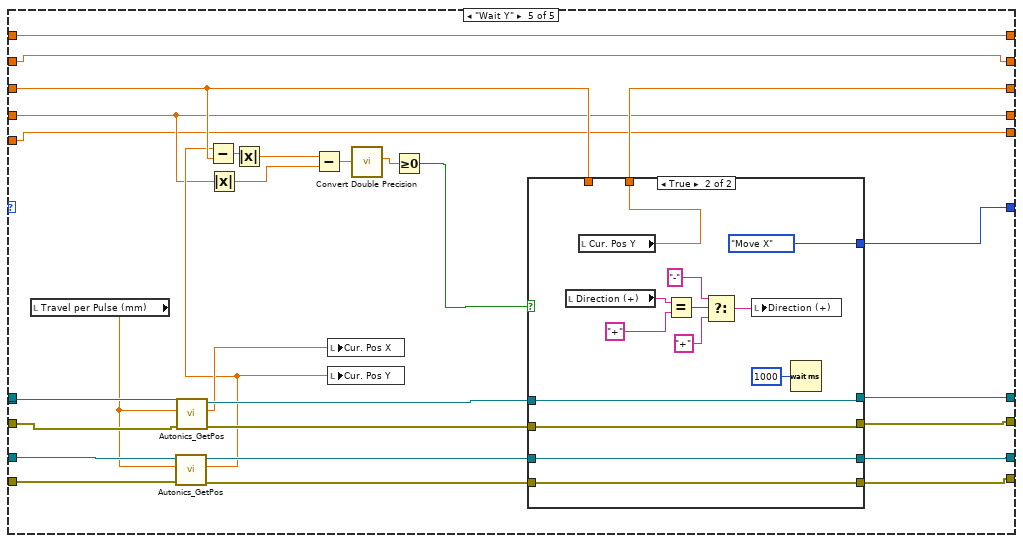
[diagram p11: hidden frame]
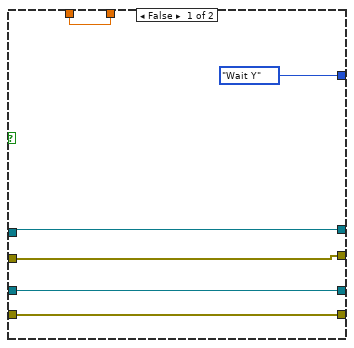
[diagram p12: hidden frame]
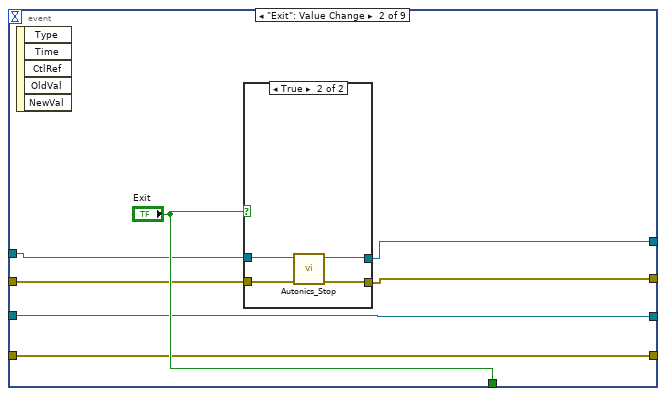
[diagram p14: hidden frame]
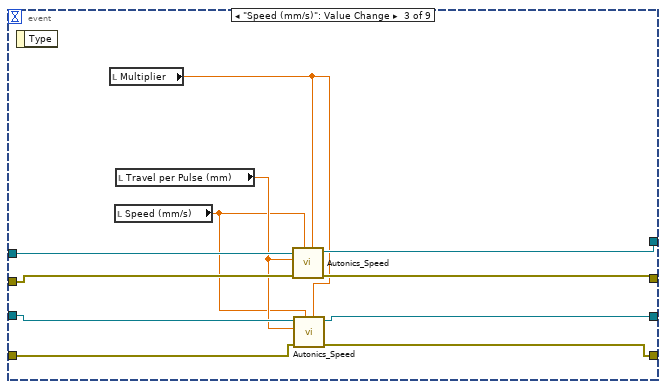
[diagram p16: hidden frame]
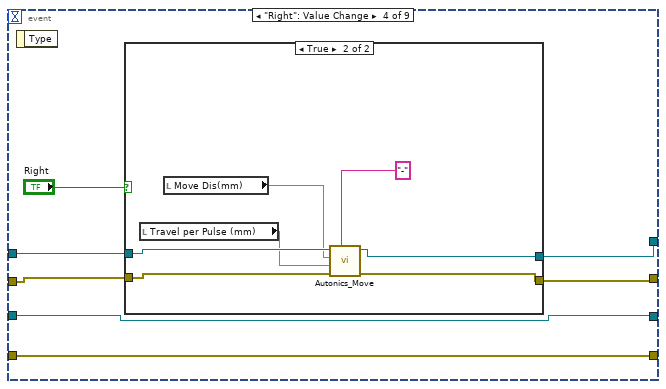
[diagram p17: hidden frame]
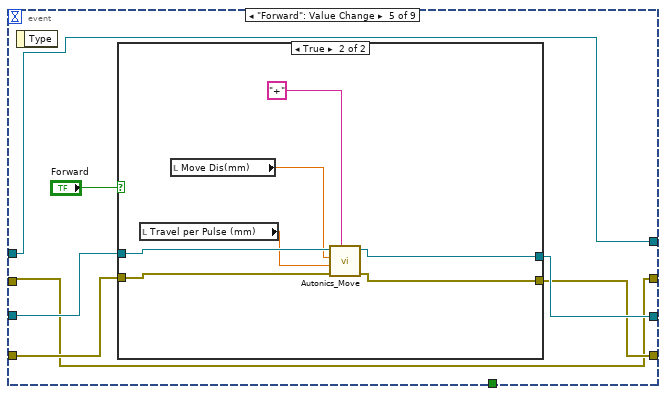
[diagram p19: hidden frame]
diagram:
  w21 = 0.0 ("Parity")
  w24 = u16 10 items=["1.0"=10, "1.5"=15, "2.0"=20] ("Stop bits")
  w25 = u16 0 items=["None", "XON/XOFF", "RTS/CTS", "XON/XOFF & RTS/CTS", "DTR/DSR", "XON/XOFF & DTR/DSR"] ("Flow control")
  w22 = u16 8 ("Data bits")
  w87 = 10178 items=["Finite Samples"=10178, "Continuous Samples"=10123, "Hardware Timed Single Point"=12522]  # Sample Mode
  # "Update. Pos X"
  # "Mov. dis Y"
  # "Old. Pos Y"
  # "Mov. dis X"
  # "Old. Pos X"
  # "div10 (Setting in Autonics controller):\n1p~0.002mm * multiplier (10)=0.02"
  # "SCANER CONTROL"
  # "1/2"
  # "start1"
  # "start2"
  # "Length"
  n1 = flat-sequence {
    tunnel: [w124] -> w67
    tunnel: [TRUE ("disable buffering (T)")] -> w49
    frame #0 {
      w100 = FALSE ("Exit")
      n2 = local write "Scan"(w100) -> ()
      n3 = local write "Exit"(w100) -> ()
    }
    frame #1 {
      n4 = disable-structure shown="Enabled" {
        frame Enabled {
          n5 = call "File Dialog"("prompt"="Choose New File For Recording\n" ("button label"), "default name"="PECT_default", "pattern (all files)"="*.tdms") -> ("selected path"=w106:path, "exists"=w102:bool, "cancelled"=w103:bool)  [unwired: 9 in, 1 out]
          n6 = case shown="False" w103 {
            tunnel: w106 -> [w107 _]
            tunnel: w102 -> [w108 _]
            frame False {
              n7 = case shown="True" w108 {
                tunnel: w107 -> [w109 w110]
                frame False {
                  n8 = local write "Record path"(w109) -> ()
                }
                frame True {
                  n9 = Two Button Dialog(message="Existing File\nDo you want to Replace?", 1:"No" ("F button name (\"Cancel\")"), 2:"Replace" ("T button name (\"OK\")")) -> (T button?=w111:bool)
                  n10 = case shown="True" w111 {
                    tunnel: w110 -> [_ w119]
                    tunnel: [path "" ("deleted path") w118] -> w112
                    frame False {
                      n11 = local write "Exit"(TRUE ("Exit")) -> ()
                    }
                    frame True {
                      n12 = Delete(path (use dialog)=w119) -> (deleted path=w118:path)  [unwired: 4 in, 2 out]
                    }
                  }
                  "Record path" <- w112
                }
              }
            }
            frame True {
              n13 = local write "Exit"(TRUE ("Exit")) -> ()
            }
          }
        }
        frame Disabled {
        }
      }
    }
    frame #2 {
      n14 = local read "Record path"() -> (w123:path)
      n15 = local write "Completed"(FALSE ("Completed")) -> ()
      n16 = TDMS Open(6:FALSE ("disable buffering (T)"), 10:T8."create or replace" ("operation"), 11:w123) -> (3:w124:refnum<k34>)  [unwired: 4 in, 1 out]
    }
  }
  n17 = local read "DAQ Pulser"() -> (w2:bool)
  n18 = call-poly <vilib>:"DAQmx Create Virtual Channel.vi"("maximum value"="Max Voltage", "minimum value"="Min Voltage", "input terminal configuration"="Terminal Configuration", "physical channels"="Physical Channel", "name to assign"="Acquisition Task") -> ("task out"=w97:refnum<k21>, "error out"=w98:errorcluster)  [unwired: 9 in]
  n19 = case shown="False" w2 {
    tunnel: ["No. Samples" w130] -> w6
    tunnel: "Sample Rate" -> [_ w131]
    frame False {
    }
    frame True {
      n20 = local read "Pulse Basic"() -> (w129:T3)
      n21 = Unbundle By Name(w129) -> ("Basic freq (Hz)"=w128:u16)
      n22 = Divide(x=w131, y=w128) -> (x/y=w132:dbl)
      n23 = Round Toward -Infinity(1:w132) -> (0:w130:dbl)
      n24 = local write "No. Samples"(w130) -> ()
    }
  }
  n25 = local read "Pulse Basic"() -> (w4:T3)
  n26 = call-poly <vilib>:"DAQmx Timing.vi"("task/channels in"=w97, "sample mode"=w87, "samples per channel"=w6, "rate"="Sample Rate", "source"="Sample Clock Source 2", "error in"=w98) -> ("task out"=w47:refnum<k21>, "error out"=w99:errorcluster)  [unwired: 8 in]
  n27 = Unbundle By Name(w4) -> ("Basic freq (Hz)"=w3:u16)
  n28 = local read "Travel per Pulse (mm)"() -> (w20:dbl)
  n29 = property class="DAQmx Timing"(reference=w47, error in=w99) -> (reference out=w45:refnum<k21>, error out=w44:errorcluster, "SampClk.Rate"=w51:dbl)
  "Actual Sample Rate" <- w51
  n30 = call-poly "VISA Configure Serial Port"("VISA resource name"="COM X", "baud rate (9600)"="Baud Rate", "data bits (8)"=w22, "parity (0:none)"=w21, "stop bits (10: 1 bit)"=w24, "flow control (0:none)"=w25) -> ("VISA resource name out"=w10:refnum<visa-resource-name>, "error out"=w11:errorcluster)  [unwired: 8 in]
  n31 = local read "Speed (mm/s)"() -> (w18:dbl)
  n32 = local read "Multiplier"() -> (w19:dbl)
  n33 = call-poly "VISA Configure Serial Port"("VISA resource name"="COM Y", "baud rate (9600)"="Baud Rate", "data bits (8)"=w22, "parity (0:none)"=w21, "stop bits (10: 1 bit)"=w24, "flow control (0:none)"=w25) -> ("VISA resource name out"=w15:refnum<visa-resource-name>, "error out"=w16:errorcluster)  [unwired: 8 in]
  n34 = call "Autonics_Speed.vi"("Multiplier"=w19, "Speed (mm/s)"=w18, "error in (no error)"=w16, "Travel per  Pulse"=w20, "VISA resource name"=w15) -> ("error out"=w29:errorcluster, "VISA resource name out"=w28:refnum<visa-resource-name>)  [unwired: 5 in]
  n35 = call "Autonics_Speed.vi"("Multiplier"="Multiplier", "Speed (mm/s)"="Speed (mm/s)", "error in (no error)"=w11, "Travel per  Pulse"="Travel per Pulse (mm)", "VISA resource name"=w10) -> ("error out"=w27:errorcluster, "VISA resource name out"=w26:refnum<visa-resource-name>)  [unwired: 5 in]
  n36 = case shown="True" "Encoder" {
    tunnel: w49 -> [_ w146]
    frame False {
    }
    frame True {
      # "Counter pulses from Motor\nto pick up signal"
      n37 = call-poly <vilib>:"DAQmx Create Virtual Channel.vi"("counter"="Motor counter") -> ("task out"=w139:refnum<k21>, "error out"=w141:errorcluster)  [unwired: 13 in]
      n38 = property class="DAQmx Channel"(reference=w139, error in=w141, "CI.CountEdges.Term"="Motor Counter Terminal") -> (reference out=w134:refnum<k21>, error out=w135:errorcluster)
      n39 = call <vilib>:"DAQmx Start Task.vi"("task/channels in"=w134, "error in"=w135) -> ("task out"=w136:refnum<k21>, "error out"=w133:errorcluster)  [unwired: 12 in]
      n40 = while {
        tunnel: w136 -> [w156]
        tunnel: w133 -> [w155]
        tunnel: [w148] -> w143
        tunnel: [w154] -> w142
        tunnel: [w147] -> _
        tunnel: w146 -> [w147]
        stop <- w149 stop-if-true
        n41 = call-poly <vilib>:"DAQmx Read.vi"("task/channels in"=w156, "error in"=w155) -> ("task out"=w154:refnum<k21>, "data"=→"Motor Pulse Count":u32, "error out"=w148:errorcluster)  [unwired: 11 in]
        n42 = Wait Until Next ms Multiple(millisecond multiple=u32 10 ("milliseconds to wait")) -> ()  [unwired: 1 out]
        n43 = local read "Completed"() -> (w150:bool)
        n44 = Unbundle By Name(w148) -> ("status"=w151:bool)
        n45 = Compound Arithmetic op=OR(w151, w150) -> (w149:bool)
      }
      n46 = call <vilib>:"DAQmx Stop Task.vi"("task/channels in"=w142, "error in"=w143) -> ("task out"=w145:refnum<k21>, "error out"=w144:errorcluster)  [unwired: 12 in]
      n47 = call <vilib>:"DAQmx Clear Task.vi"("task in"=w145, "error in"=w144) -> ("error out"=w137:errorcluster)  [unwired: 13 in]
      n48 = call <vilib>:"Simple Error Handler.vi"("error in (no error)"=w137) -> ()  [unwired: 4 in, 5 out]
    }
  }
  n49 = while {
    shift-right: [w169] -> w40
    shift-left: w26 -> [w168]
    shift-right: [w159] -> w39
    shift-left: w27 -> [w167]
    shift-right: [w162] -> w41
    shift-left: w28 -> [w164]
    shift-right: [w161] -> w42
    shift-left: w29 -> [w163]
    stop <- w166 stop-if-true
    n50 = event shown="[0] Timeout" {
      selector: _ -> [_ _ _ _ _ _ _ _ _]
      dyn-events: _ -> [_ _ _ _ _ _ _ _ _]
      timeout: 100 -> [_ _ _ _ _ _ _ _ _]
      tunnel: w168 -> [w177 w199 w217 w222 w234 w254 w267 w290 w317]
      tunnel: w167 -> [w176 w198 w216 w221 w235 w253 w266 w289 w316]
      tunnel: [w173 w197 w215 w224 w234 w256 w267 w287 w319] -> w169
      tunnel: [w172 w196 w214 w223 w235 w255 w266 w286 w318] -> w159
      tunnel: [_ "Exit" _ _ _ _ _ _ _] -> w165
      tunnel: w164 -> [w175 w194 w213 w219 w239 w251 w270 w285 w314]
      tunnel: w163 -> [w174 w195 w210 w218 w238 w250 w271 w284 w312]
      tunnel: [w171 w194 w212 w219 w237 w251 w268 w282 w313] -> w162
      tunnel: [w170 w195 w211 w218 w236 w250 w269 w283 w311] -> w161
      event Timeout {
        n51 = event-data() -> ()  [unwired: 1 in, 1 out]
        n52 = local read "Scan"() -> (w178:bool)
        n53 = case shown="False" w178 {
          tunnel: w175 -> [w189 w191]
          tunnel: w174 -> [w188 w190]
          tunnel: [w187 w191] -> w171
          tunnel: [w186 w190] -> w170
          tunnel: w176 -> [w185 w192]
          tunnel: w177 -> [w184 w193]
          tunnel: [w183 w193] -> w173
          tunnel: [w182 w192] -> w172
          frame False {
            n54 = local read "Travel per Pulse (mm)"() -> (w181:dbl)
            n55 = call "Autonics_GetPos.vi"("error in (no error)"=w188, "Travel per Pulse (mm)"=w181, "VISA resource name"=w189) -> ("error out"=w186:errorcluster, "Current  Position (mm)"=w179:dbl, "VISA resource name out"=w187:refnum<visa-resource-name>)  [unwired: 6 in]
            n56 = call "Autonics_GetPos.vi"("error in (no error)"=w185, "Travel per Pulse (mm)"=w181, "VISA resource name"=w184) -> ("error out"=w182:errorcluster, "Current  Position (mm)"=w180:dbl, "VISA resource name out"=w183:refnum<visa-resource-name>)  [unwired: 6 in]
            n57 = local write "Cur. Pos Y"(w179) -> ()
            n58 = local write "Cur. Pos X"(w180) -> ()
          }
          frame True {
          }
        }
      }
      event "Exit": Value Change {
        n59 = event-data() -> ()  [unwired: 1 in, 5 out]
        n60 = case shown="True" "Exit" {
          tunnel: [w202 w205] -> w197
          tunnel: [w201 w206] -> w196
          tunnel: w199 -> [w202 w204]
          tunnel: w198 -> [w201 w203]
          frame False {
          }
          frame True {
            n61 = call "Autonics_Stop.vi"("error in (no error)"=w203, "VISA resource name"=w204) -> ("error out"=w206:errorcluster, "VISA resource name out"=w205:refnum<visa-resource-name>)  [unwired: 8 in]
          }
        }
      }
      event "Speed (mm/s)": Value Change {
        n62 = event-data() -> ()  [unwired: 1 in, 1 out]
        n63 = local read "Multiplier"() -> (w207:dbl)
        n64 = local read "Speed (mm/s)"() -> (w208:dbl)
        n65 = local read "Travel per Pulse (mm)"() -> (w209:dbl)
        n66 = call "Autonics_Speed.vi"("Multiplier"=w207, "Speed (mm/s)"=w208, "error in (no error)"=w216, "Travel per  Pulse"=w209, "VISA resource name"=w217) -> ("error out"=w214:errorcluster, "VISA resource name out"=w215:refnum<visa-resource-name>)  [unwired: 5 in]
        n67 = call "Autonics_Speed.vi"("Multiplier"=w207, "Speed (mm/s)"=w208, "error in (no error)"=w210, "Travel per  Pulse"=w209, "VISA resource name"=w213) -> ("error out"=w211:errorcluster, "VISA resource name out"=w212:refnum<visa-resource-name>)  [unwired: 5 in]
      }
      event "Right": Value Change {
        n68 = event-data() -> ()  [unwired: 1 in, 1 out]
        n69 = case shown="True" "Right" {
          tunnel: [w225 w231] -> w224
          tunnel: [w226 w227] -> w223
          tunnel: w222 -> [w225 w233]
          tunnel: w221 -> [w226 w232]
          frame False {
          }
          frame True {
            n70 = local read "Travel per Pulse (mm)"() -> (w229:dbl)
            n71 = local read "Move Dis(mm)"() -> (w230:dbl)
            n72 = call "Autonics_Move.vi"("Direction (+)"="-", "error in (no error)"=w232, "Travel per Pulse (mm)"=w229, "Move Distance (mm)"=w230, "VISA resource name"=w233) -> ("error out"=w227:errorcluster, "VISA resource name out"=w231:refnum<visa-resource-name>)  [unwired: 5 in]
          }
        }
      }
      event "Forward": Value Change {
        n73 = event-data() -> ()  [unwired: 1 in, 1 out]
        n74 = case shown="True" "Forward" {
          tunnel: [w241 w247] -> w237
          tunnel: [w242 w246] -> w236
          tunnel: w239 -> [w241 w249]
          tunnel: w238 -> [w242 w248]
          frame False {
          }
          frame True {
            n75 = local read "Travel per Pulse (mm)"() -> (w244:dbl)
            n76 = local read "Move Dis(mm)"() -> (w245:dbl)
            n77 = call "Autonics_Move.vi"("Direction (+)"="+", "error in (no error)"=w248, "Travel per Pulse (mm)"=w244, "Move Distance (mm)"=w245, "VISA resource name"=w249) -> ("error out"=w246:errorcluster, "VISA resource name out"=w247:refnum<visa-resource-name>)  [unwired: 5 in]
          }
        }
      }
      event "Left": Value Change {
        n78 = event-data() -> ()  [unwired: 1 in, 1 out]
        n79 = case shown="True" "Left" {
          tunnel: [w258 w263] -> w256
          tunnel: [w257 w262] -> w255
          tunnel: w254 -> [w258 w265]
          tunnel: w253 -> [w257 w264]
          frame False {
          }
          frame True {
            # "Moving distance"
            n80 = local read "Travel per Pulse (mm)"() -> (w259:dbl)
            n81 = local read "Move Dis(mm)"() -> (w260:dbl)
            n82 = call "Autonics_Move.vi"("Direction (+)"="+", "error in (no error)"=w264, "Travel per Pulse (mm)"=w259, "Move Distance (mm)"=w260, "VISA resource name"=w265) -> ("error out"=w262:errorcluster, "VISA resource name out"=w263:refnum<visa-resource-name>)  [unwired: 5 in]
          }
        }
      }
      event "Backward": Value Change {
        n83 = event-data() -> ()  [unwired: 1 in, 1 out]
        n84 = case shown="True" "Backward" {
          tunnel: [w274 w279] -> w268
          tunnel: [w273 w278] -> w269
          tunnel: w270 -> [w274 w281]
          tunnel: w271 -> [w273 w280]
          frame False {
          }
          frame True {
            # "Moving distance"
            n85 = local read "Travel per Pulse (mm)"() -> (w275:dbl)
            n86 = local read "Move Dis(mm)"() -> (w276:dbl)
            n87 = call "Autonics_Move.vi"("Direction (+)"="-", "error in (no error)"=w280, "Travel per Pulse (mm)"=w275, "Move Distance (mm)"=w276, "VISA resource name"=w281) -> ("error out"=w278:errorcluster, "VISA resource name out"=w279:refnum<visa-resource-name>)  [unwired: 5 in]
          }
        }
      }
      event "Home": Value Change {
        n88 = event-data() -> ()  [unwired: 1 in, 1 out]
        n89 = case shown="True" "Home" {
          tunnel: [w294 w306] -> w287
          tunnel: [w293 w305] -> w286
          tunnel: w290 -> [w294 w310]
          tunnel: w289 -> [w293 w309]
          tunnel: w285 -> [w292 w302]
          tunnel: w284 -> [w291 w301]
          tunnel: [w292 w300] -> w282
          tunnel: [w291 w299] -> w283
          frame False {
          }
          frame True {
            n90 = call "Autonics_Home.vi"("error in (no error)"=w309, "VISA resource name"=w310) -> ("error out"=w307:errorcluster, "VISA resource name out"=w308:refnum<visa-resource-name>)  [unwired: 8 in]
            n91 = call "Autonics_Home.vi"("error in (no error)"=w301, "VISA resource name"=w302) -> ("error out"=w304:errorcluster, "VISA resource name out"=w303:refnum<visa-resource-name>)  [unwired: 8 in]
            n92 = local read "Travel per Pulse (mm)"() -> (w298:dbl)
            n93 = local read "Speed (mm/s)"() -> (w297:dbl)
            n94 = local read "Multiplier"() -> (w296:dbl)
            n95 = local write "Home"(FALSE ("Home")) -> ()
            n96 = call "Autonics_Speed.vi"("Multiplier"=w296, "Speed (mm/s)"=w297, "error in (no error)"=w307, "Travel per  Pulse"=w298, "VISA resource name"=w308) -> ("error out"=w305:errorcluster, "VISA resource name out"=w306:refnum<visa-resource-name>)  [unwired: 5 in]
            n97 = call "Autonics_Speed.vi"("Multiplier"=w296, "Speed (mm/s)"=w297, "error in (no error)"=w304, "Travel per  Pulse"=w298, "VISA resource name"=w303) -> ("error out"=w299:errorcluster, "VISA resource name out"=w300:refnum<visa-resource-name>)  [unwired: 5 in]
          }
        }
      }
      event "Stop": Value Change {
        n98 = event-data() -> ()  [unwired: 1 in, 1 out]
        n99 = case shown="False" "Stop" {
          tunnel: [w321 w328] -> w319
          tunnel: [w323 w331] -> w318
          tunnel: w317 -> [w321 w330]
          tunnel: w316 -> [w323 w329]
          tunnel: w314 -> [w322 w327]
          tunnel: [w322 w326] -> w313
          tunnel: w312 -> [w320 w325]
          tunnel: [w320 w324] -> w311
          frame False {
          }
          frame True {
            n100 = call "Autonics_Stop.vi"("error in (no error)"=w329, "VISA resource name"=w330) -> ("error out"=w331:errorcluster, "VISA resource name out"=w328:refnum<visa-resource-name>)  [unwired: 8 in]
            n101 = call "Autonics_Stop.vi"("error in (no error)"=w325, "VISA resource name"=w327) -> ("error out"=w324:errorcluster, "VISA resource name out"=w326:refnum<visa-resource-name>)  [unwired: 8 in]
          }
        }
      }
    }
    n102 = Unbundle By Name(w161) -> ("status"=w160:bool)
    n103 = Unbundle By Name(w159) -> ("status"=w158:bool)
    n104 = Compound Arithmetic op=OR(w160, w165, w158) -> (w166:bool)
  }
  n105 = call-poly <vilib>:"DAQmx Trigger.vi"("task/channels in"=w45, "source"="Pulser Trigger", "edge"="Edge", "error in"=w44) -> ("task out"=w84:refnum<k21>, "error out"=w83:errorcluster)  [unwired: 10 in]
  n106 = local read "Y - length"() -> (w8:dbl)
  n107 = property class="DAQmx Trigger"(reference=w84, error in=w83, "Start.Retriggerable"=TRUE) -> (reference out=w69:refnum<k21>, error out=w50:errorcluster)
  n108 = case shown="True" "DAQ Pulser" {
    tunnel: w50 -> [_ w362]
    frame False {
    }
    frame True {
      (unwired) 1 ("x")
      w359 = 10123 items=["Finite Samples"=10178, "Continuous Samples"=10123, "Hardware Timed Single Point"=12522]  # Sample Mode
      n109 = local read "Pulse Basic"() -> (w333:T3)
      n110 = Unbundle By Name(w333) -> ("Basic freq (Hz)"=w332:u16)
      n111 = call-poly <vilib>:"DAQmx Create Virtual Channel.vi"("maximum value"="Max Voltage 2", "minimum value"="Min Voltage 2", "physical channels"="Physical Channel(s)", "name to assign"="Pulser Task", "error in"=w362) -> ("task out"=w353:refnum<k21>, "error out"=w352:errorcluster)  [unwired: 9 in]
      n112 = Divide(x="Sample Rate 2", y=w332) -> (x/y=w350:dbl)
      n113 = Multiply(x="Pulser Cycles", y=w350) -> (x*y=w349:dbl)
      n114 = Round Toward -Infinity(1:w349) -> (0:w341:dbl)
      "Sample per Channel AO" <- w341
      n115 = call-poly <vilib>:"DAQmx Timing.vi"("task/channels in"=w353, "sample mode"=w359, "samples per channel"=w341, "rate"="Sample Rate 2", "source"="Sample Clock Source", "error in"=w352) -> ("task out"=w361:refnum<k21>, "error out"=w360:errorcluster)  [unwired: 8 in]
      n116 = property class="DAQmx Timing"(reference=w361, error in=w360) -> (reference out=w348:refnum<k21>, error out=w334:errorcluster, "SampClk.Rate"=w336:dbl)
      "Actual Sample Rate 2" <- w336
      n117 = call "waveform_generator.vi"("Sampling rate"=w336, "Pulse chirp"="Pulse chirp", "Pulse Gaussian"="Pulse Gaussian", "Cluster Basic"="Pulse Basic", "Tab Control"="Tab Control 4") -> ("Waveform Graph"=w335:waveform(dbl)[])  [unwired: 6 in]
      n118 = disable-structure shown="Enabled" {
        disable-tunnel: w335 -> [w367 w388]
        disable-tunnel: [w366 w391] -> w345
        disable-tunnel: [w365 w390] -> w342
        disable-tunnel: w348 -> [w364 w392]
        disable-tunnel: w334 -> [w363 w387]
        frame Disabled {
          n119 = while {
            tunnel: w367 -> [w378]
            shift-right: [w374] -> w366
            shift-left: w364 -> [w372]
            shift-right: [w373] -> w365
            shift-left: w363 -> [w371]
            stop <- FALSE stop-if-true
            n120 = call-poly <vilib>:"DAQmx Write.vi"("task/channels in"=w372, "data"=w378, "timeout"=-1.0, "error in"=w371) -> ("task out"=w377:refnum<k21>, "error out"=w376:errorcluster)  [unwired: 9 in, 1 out]
            n121 = call <vilib>:"DAQmx Start Task.vi"("task/channels in"=w377, "error in"=w376) -> ("task out"=w370:refnum<k21>, "error out"=w369:errorcluster)  [unwired: 12 in]
            n122 = disable-structure shown="Enabled" {
              disable-tunnel: [w384 w386] -> w374
              disable-tunnel: [w383 w385] -> w373
              disable-tunnel: w370 -> [w382 w386]
              disable-tunnel: w369 -> [w381 w385]
              frame Disabled {
                n123 = call <vilib>:"DAQmx Wait Until Done.vi"("task/channels in"=w382, "error in"=w381) -> ("task out"=w380:refnum<k21>, "error out"=w379:errorcluster)  [unwired: 12 in]
                n124 = call <vilib>:"DAQmx Stop Task.vi"("task/channels in"=w380, "error in"=w379) -> ("task out"=w384:refnum<k21>, "error out"=w383:errorcluster)  [unwired: 12 in]
              }
              frame Enabled {
              }
            }
          }
        }
        frame Enabled {
          n125 = call-poly <vilib>:"DAQmx Write.vi"("task/channels in"=w392, "data"=w388, "timeout"=-1.0, "error in"=w387) -> ("task out"=w394:refnum<k21>, "error out"=w396:errorcluster)  [unwired: 9 in, 1 out]
          n126 = call <vilib>:"DAQmx Start Task.vi"("task/channels in"=w394, "error in"=w396) -> ("task out"=w393:refnum<k21>, "error out"=w395:errorcluster)  [unwired: 12 in]
          n127 = while {
            tunnel: w393 -> [w404]
            tunnel: w395 -> [w403]
            tunnel: [w401] -> w390
            tunnel: [w402] -> w391
            stop <- w398 stop-if-true
            n128 = call <vilib>:"DAQmx Is Task Done.vi"("task/channels in"=w404, "error in"=w403) -> ("task out"=w402:refnum<k21>, "error out"=w401:errorcluster)  [unwired: 11 in, 1 out]
            n129 = Unbundle By Name(w401) -> ("status"=w399:bool)
            n130 = local read "Exit"() -> (w397:bool)
            n131 = Wait Until Next ms Multiple(millisecond multiple=u32 100) -> ()  [unwired: 1 out]
            n132 = Compound Arithmetic op=OR(w399, w397) -> (w398:bool)
          }
        }
      }
      n133 = call <vilib>:"DAQmx Stop Task.vi"("task/channels in"=w345, "error in"=w342) -> ("task out"=w344:refnum<k21>, "error out"=w343:errorcluster)  [unwired: 12 in]
      n134 = call <vilib>:"DAQmx Clear Task.vi"("task in"=w344, "error in"=w343) -> ("error out"=w358:errorcluster)  [unwired: 13 in]
      n135 = call <vilib>:"Simple Error Handler.vi"("error in (no error)"=w358) -> ()  [unwired: 4 in, 5 out]
    }
  }
  n136 = local read "X - length"() -> (w74:dbl)
  n137 = local read "Step Y"() -> (w72:dbl)
  n138 = local read "Step X"() -> (w73:dbl)
  n139 = Quotient & Remainder(x=w8, y=w72) -> (floor(x/y)=w48:dbl)  [unwired: 1 out]
  n140 = Quotient & Remainder(x=w74, y=w73) -> (floor(x/y)=w65:dbl)  [unwired: 1 out]
  n141 = Obtain Queue(max queue size (-1, unlimited)=10000, name (unnamed)="data DAQ", element data type=dbl[] [] ("data")) -> (queue out=w79:refnum<queue>)  [unwired: 2 in, 2 out]
  n142 = Increment(x=w48) -> (x+1=w7:dbl)
  n143 = Build Array(w3, w51, w65, w7) -> (w56:dbl[])
  n144 = TDMS Write(0:w67, 5:"Freq_Sampling_SizeX_SizeY" ("group name in (Untitled)"), 9:w56) -> (4:w66:refnum<k34>)  [unwired: 3 in, 3 out]
  n145 = call "PECT_GateConverse.vi"("Gate 2"="Gate 2", "Gate 1"="Gate 1", "Freq_Sampling_SizeX_SizeY"=w56) -> ("Length T/2"=w57:i32, "Length"=w58:i32, "Start 2"=w59:i32, "Start 1"=w60:i32)  [unwired: 4 in, 1 out]
  n146 = Initialize Array(0.0 ("element"), w6) -> (w80:dbl[])
  n147 = Obtain Queue(name (unnamed)="data Extraction", element data type=0.0) -> (queue out=w77:refnum<queue>)  [unwired: 3 in, 2 out]
  n148 = Obtain Queue(max queue size (-1, unlimited)=2 ("최대 큐 크기(-1,제한없음)"), name (unnamed)="2D data", element data type=dbl[][] [] ("initialized array")) -> (queue out=w53:refnum<queue>)  [unwired: 2 in, 2 out]
  n149 = case shown="\"                    Test mode                   \"" "Tab Control 2" {
    tunnel: w69 -> [w443 w699 w725]
    tunnel: [w442 w699 w724] -> w90
    tunnel: [w441 w698 w723] -> w89
    tunnel: w80 -> [w438 _ w722]
    tunnel: w50 -> [w440 w698 w721]
    tunnel: w57 -> [w439 _ w720]
    tunnel: w79 -> [w437 _ _]
    tunnel: w77 -> [w416 _ _]
    tunnel: w65 -> [w412 _ _]
    tunnel: w7 -> [w413 _ _]
    tunnel: w58 -> [w424 _ w718]
    tunnel: w60 -> [w423 _ w717]
    tunnel: w59 -> [w422 _ w716]
    tunnel: w66 -> [w421 _ _]
    tunnel: "Waveform" ("group name in (Untitled)") -> [w418 _ _]
    tunnel: w53 -> [w414 _ _]
    tunnel: w6 -> [w409 _ w715]
    frame "                          Scan mode                      ", Default {
      # "Column"
      # "Row"
      n150 = Initialize Array(0.0 ("element"), w412, w413) -> (w430:dbl[][])
      n151 = local read "3D Surface"() -> (w425:refnum<k7>)
      n152 = Matrix Size(0:w430) -> (1:w431:i32, 2:w432:i32)
      n153 = local read "Step X"() -> (w407:dbl)
      n154 = Decrement(x=w431) -> (x-1=w435:i32)
      n155 = Decrement(x=w432) -> (x-1=w434:i32)
      n156 = call "Surface_AxesScale.vi"("Y-axis Max"=w434, "X-axis max"=w435, "3D Surface"=w425, "Auto Scale"=FALSE) -> ()  [unwired: 8 in]
      n157 = Multiply(x=w407, y=-10) -> (x*y=w406:dbl)
      n158 = To Long Integer(number=w406) -> (32bit integer=w405:i32)
      n159 = while {
        shift-right: [w489] -> _
        shift-left: 0 -> [w491]
        shift-right: [w488] -> _
        shift-left: 0 -> [w490]
        tunnel: w416 -> [w487]
        shift-right: [w479] -> w410
        shift-left: w430 -> [w486]
        shift-right: [w482] -> _
        shift-left: TRUE ("Output Direction") -> [w483]
        tunnel: w414 -> [w481]
        tunnel: [w480] -> w415
        stop <- w484 stop-if-true
        n160 = local read "Scan"() -> (w478:bool)
        n161 = local read "Completed"() -> (w477:bool)
        n162 = Compound Arithmetic op=AND(invert w478, invert w477) -> (w476:bool)
        n163 = case shown="False" w476 {
          tunnel: w491 -> [w508 w554]
          tunnel: w490 -> [w507 w553]
          tunnel: [w506 w554] -> w489
          tunnel: [w500 w553] -> w488
          tunnel: w487 -> [w505 w546]
          tunnel: w486 -> [w504 w550]
          tunnel: [w497 w533] -> w479
          tunnel: [w503 _] -> w475
          tunnel: w483 -> [w502 w552]
          tunnel: [w501 w552] -> w482
          tunnel: w481 -> [w498 w535]
          tunnel: [w496 w546] -> w480
          frame False {
            n164 = Dequeue Element(queue=w505, timeout in ms (-1)=5000) -> (queue out=w496:refnum<queue>, element=w499:dbl)  [unwired: 1 in, 2 out]
            n165 = call "EletoMatr_1channel.vi"("Input Array X"=w504, "Input data"=w499, "In Row"=w508, "In Column"=w507, "Input Direction"=w502) -> ("Completed"=w503:bool, "Out Array X"=w497:dbl[][], "Out Row"=w506:i32, "Output Direction"=w501:bool, "Out Column"=w500:i32)  [unwired: 6 in]
            n166 = Lossy Enqueue Element(queue=w498, element=w497) -> ()  [unwired: 1 in, 4 out]
          }
          frame True {
            n167 = local read "Gate 1"() -> (w549:dbl)
            n168 = local read "Gate 2"() -> (w548:dbl)
            n169 = Wait Until Next ms Multiple(millisecond multiple=u32 100 ("ms 배수")) -> ()  [unwired: 1 out]
            n170 = local read "Offset"() -> (w540:bool)
            n171 = call "TDMS_Open.vi"("Offset"=w540, "Gate 2"=w548, "Gate 1"=w549, "Input 2D"=w550, "Open"="Open tdms") -> ("Output 2D"=w513:dbl[][])  [unwired: 5 in, 1 out]
            n172 = case shown="True" "Open tdms" {
              tunnel: w513 -> [_ w555]
              frame False {
              }
              frame True {
                n173 = global write "Global_data.vi" "global 2d graph"(w555) -> ()
              }
            }
            n174 = call "RepairLine.vi"("Repair Line Col"="Repair Line Col", "Repair Line Row"="Repair Line Row", "Line Col"="Line Col", "Line Row"="Line Row", "Array In"=w513) -> ("Array Repaired"=w527:dbl[][])  [unwired: 6 in]
            n175 = call "CSV Open.vi"("2D Array In"=w527, "Open"="Open csv") -> ("2D Array Out"=w534:dbl[][])  [unwired: 9 in]
            n176 = call "Backdata.vi"("Backindex"="Backindex", "Array in"=w534, "Backdata"="Backdata") -> ("Array out"=w516:dbl[][])
            n177 = call "TrimXY.vi"("X-max"="Y-max", "X-min"="Y-min", "Y-max"="X-max", "Y-min"="X-min", "Array In"=w516, "Trim data"="Trim data") -> ("Array Trim Out"=w515:dbl[][])  [unwired: 5 in]
            n178 = global read "Global_data.vi" "global 2d graph"() -> (w510:dbl[][])
            n179 = call "Inverse.vi"(10:"Inverse"=w515, 11:"Inverse"="Inverse") -> ("Array out"=w511:dbl[][])  [unwired: 9 in]
            n180 = call "Return data.vi"("Array Return"=w510, "Array Input"=w511, "Return"="Return") -> ("Array out"=w509:dbl[][])  [unwired: 8 in]
            n181 = call "Abs.vi"("Input"=w509, "Abs"="Abs") -> ("Array out"=w539:dbl[][])  [unwired: 9 in]
            n182 = call "DiffX.vi"("Array in"=w539, "DiffX"="DiffX") -> ("Array out"=w544:dbl[][])  [unwired: 1 in]
            n183 = call "DiffY.vi"("Array in"=w544, "DiffY"="DiffY") -> ("Array out"=w542:dbl[][])  [unwired: 1 in]
            n184 = call "Odd.vi"("Odd"="Odd", "Array In"=w542) -> ("Array Out"=w531:dbl[][])  [unwired: 9 in]
            n185 = call "Filter_Lowpass - 2D.vi"("Filter"="Filter", "Input 2D"=w531, "low cutoff freq: fl"="low cutoff freq: fl") -> ("Output"=w530:dbl[][])  [unwired: 6 in]
            n186 = case shown="True" TRUE {
              tunnel: w530 -> [w556 w557]
              tunnel: [w556 w557] -> w533
              tunnel: w535 -> [_ w558]
              frame False {
              }
              frame True {
                n187 = local read "3D Surface"() -> (w562:refnum<k7>)
                n188 = Matrix Size(0:w557) -> (1:w563:i32, 2:w560:i32)
                n189 = Decrement(x=w563) -> (x-1=w561:i32)
                n190 = Decrement(x=w560) -> (x-1=w559:i32)
                n191 = call "Surface_AxesScale.vi"("Y-axis Max"=w559, "X-axis max"=w561, "3D Surface"=w562, "Auto Scale"=FALSE) -> ()  [unwired: 8 in]
                n192 = Lossy Enqueue Element(queue=w558, element=w557) -> ()  [unwired: 1 in, 4 out]
              }
            }
          }
        }
        "Output" <- w479
        n193 = case shown="True" w475 {
          selector: w475 -> [w492 w493]
          tunnel: [w492 w493] -> w474
          frame False {
          }
          frame True {
            n194 = Wait (ms)(milliseconds to wait=u32 200) -> ()  [unwired: 1 out]
          }
        }
        "Completed" <- w474
        n195 = local read "Exit"() -> (w485:bool)
        n196 = Compound Arithmetic op=OR(w474, w485) -> (w484:bool)
        "No. Y" <- w490
        "No. X" <- w491
      }
      n197 = while {
        tunnel: w443 -> [w574]
        tunnel: [w573] -> w442
        tunnel: [w572] -> w441
        tunnel: w440 -> [w571]
        tunnel: w437 -> [w570]
        tunnel: w409 -> [w565]
        stop <- w566 stop-if-true
        n198 = case shown="True" "Scan" {
          tunnel: w574 -> [w576 w582]
          tunnel: [w576 w581] -> w573
          tunnel: [w575 w580] -> w572
          tunnel: w571 -> [w575 w579]
          tunnel: w570 -> [_ w578]
          tunnel: w565 -> [_ w577]
          frame False {
          }
          frame True {
            n199 = while {
              tunnel: w582 -> [w596]
              tunnel: [w599] -> w581
              tunnel: [w598] -> w580
              tunnel: w579 -> [w595]
              tunnel: w578 -> [w597]
              tunnel: w577 -> [w587]
              stop <- w588 stop-if-true
              n200 = First Call?() -> (First Call?: T/F=w592:bool)
              n201 = case shown="True" w592 {
                tunnel: w596 -> [w600 w605]
                tunnel: w595 -> [w601 w604]
                tunnel: [w600 w603] -> w594
                tunnel: [w601 w602] -> w593
                frame False {
                }
                frame True {
                  n202 = call <vilib>:"DAQmx Start Task.vi"("task/channels in"=w605, "error in"=w604) -> ("task out"=w603:refnum<k21>, "error out"=w602:errorcluster)  [unwired: 12 in]
                }
              }
              n203 = call-poly <vilib>:"DAQmx Read.vi"("task/channels in"=w594, "timeout"=w587, "error in"=w593) -> ("task out"=w599:refnum<k21>, "data"=w585:waveform(dbl)[], "error out"=w598:errorcluster)  [unwired: 10 in]
              n204 = Index Array(array=w585, index=0 ("index (row)")) -> (element=w584:waveform(dbl))
              n205 = Unbundle By Name(w584) -> ("Y"=w583:dbl[])
              n206 = Enqueue Element(queue=w597, element=w583) -> ()  [unwired: 2 in, 3 out]
              n207 = Unbundle By Name(w598) -> ("status"=w589:bool)
              n208 = local read "Completed"() -> (w591:bool)
              n209 = local read "Exit"() -> (w590:bool)
              n210 = Compound Arithmetic op=OR(w589, w591, w590) -> (w588:bool)
            }
          }
        }
        n211 = local read "Completed"() -> (w567:bool)
        n212 = local read "Exit"() -> (w568:bool)
        n213 = Compound Arithmetic op=OR(w567, w568) -> (w566:bool)
      }
      n214 = while {
        shift-right: [w622] -> _
        shift-left: w438 -> [w626]
        tunnel: w438 -> [w625]
        tunnel: w439 -> [w624]
        tunnel: w437 -> [w623]
        tunnel: w416 -> [w621]
        shift-right: [w618] -> _
        shift-left: 0 -> [w619]
        tunnel: w424 -> [w617]
        tunnel: w423 -> [w616]
        tunnel: w422 -> [w615]
        tunnel: w421 -> [w614]
        tunnel: [w613] -> w420
        tunnel: [w612] -> w419
        tunnel: w418 -> [w611]
        shift-right: [w609] -> _
        shift-left: w405 -> [w610]
        stop <- w606 stop-if-true
        n215 = local read "Scan"() -> (w620:bool)
        n216 = case shown="True" w620 {
          tunnel: w626 -> [w631 w644]
          tunnel: w625 -> [_ w650]
          tunnel: w624 -> [_ w649]
          tunnel: w623 -> [_ w648]
          tunnel: [w631 w647] -> w622
          tunnel: w621 -> [_ w646]
          tunnel: w619 -> [w630 w642]
          tunnel: [w630 w641] -> w618
          tunnel: w617 -> [_ w640]
          tunnel: w616 -> [_ w639]
          tunnel: w615 -> [_ w638]
          tunnel: w614 -> [w628 w637]
          tunnel: [w628 w636] -> w613
          tunnel: [_ w635] -> w612
          tunnel: w611 -> [_ w634]
          tunnel: w610 -> [w627 w633]
          tunnel: [w627 w632] -> w609
          frame False {
            n217 = Wait Until Next ms Multiple(millisecond multiple=u32 100 ("ms 배수")) -> ()  [unwired: 1 out]
          }
          frame True {
            n218 = local read "Pulser Cycles"() -> (w643:i32)
            n219 = Increment(x=w642) -> (x+1=w641:i32)
            n220 = Dequeue Element(queue=w648) -> (element=w645:dbl[])  [unwired: 2 in, 3 out]
            n221 = Quotient & Remainder(x=w641, y=w643) -> (x-y*floor(x/y)=w651:i32)  [unwired: 1 out]
            n222 = Add(x=w645, y=w644) -> (x+y=w653:dbl[])
            n223 = Equal To 0?(x=w651) -> (x = 0?=w652:bool)
            n224 = case shown="True" w652 {
              tunnel: w643 -> [_ w675]
              tunnel: w653 -> [w656 w673]
              tunnel: [w656 w676] -> w647
              tunnel: w650 -> [_ w676]
              tunnel: w649 -> [_ w669]
              tunnel: w646 -> [_ w674]
              tunnel: w640 -> [_ w670]
              tunnel: w639 -> [_ w672]
              tunnel: w638 -> [_ w671]
              tunnel: w637 -> [w655 w663]
              tunnel: [w655 w661] -> w636
              tunnel: [_ w660] -> w635
              tunnel: w634 -> [_ w662]
              tunnel: w633 -> [w654 w665]
              tunnel: [w654 w664] -> w632
              frame False {
                n225 = disable-structure shown="비활성화" {
                  frame Disabled {
                    n226 = Wait Until Next ms Multiple(millisecond multiple=u32 100 ("ms 배수")) -> ()  [unwired: 1 out]
                  }
                  frame Enabled {
                  }
                }
              }
              frame True {
                n227 = local read "Encoder"() -> (w658:bool)
                n228 = Divide(x=w673, y=w675) -> (x/y=w659:dbl[])
                n229 = case shown="True" w658 {
                  tunnel: [w678 w682] -> w666
                  tunnel: w665 -> [w677 w679]
                  tunnel: [w677 w680] -> w664
                  frame False {
                    n230 = local read "Acquire"() -> (w678:bool)
                  }
                  frame True {
                    n231 = local read "Motor Pulse Count"() -> (w681:i32)
                    n232 = local read "Step X"() -> (w687:dbl)
                    n233 = Multiply(x=w687, y=10) -> (x*y=w685:dbl)
                    n234 = To Long Integer(number=w685) -> (32bit integer=w684:i32)
                    n235 = Add(x=w684, y=w679) -> (x+y=w683:i32)
                    n236 = Greater Or Equal?(x=w681, y=w683) -> (x >= y?=w682:bool)
                    "x <= y?" <- w682
                    n237 = Select(t=w681, s=w682, f=w679) -> (s? t:f=w680:i32)
                  }
                }
                n238 = local read "Offset"() -> (w668:bool)
                n239 = call "PECT_Feature extraction.vi"("Length T/2"=w669, "Offset"=w668, "Length"=w670, "Start 2"=w671, "Start 1"=w672, "Pulse signal in"=w659) -> ("Feature extraction out"=w667:dbl)  [unwired: 5 in]
                n240 = case shown="True" w666 {
                  tunnel: w674 -> [_ w696]
                  tunnel: w667 -> [_ w695]
                  tunnel: w663 -> [w688 w694]
                  tunnel: w662 -> [_ w693]
                  tunnel: w659 -> [_ w689]
                  tunnel: [w688 w692] -> w661
                  tunnel: [_ w691] -> w660
                  frame False {
                  }
                  frame True {
                    n241 = TDMS Write(0:w694, 5:w693, 9:w689) -> (4:w692:refnum<k34>, 15:w691:errorcluster)  [unwired: 3 in, 2 out]
                    n242 = Enqueue Element(queue=w696, element=w695) -> ()  [unwired: 2 in, 3 out]
                    n243 = local write "Acquire"(FALSE ("Acquire")) -> ()
                  }
                }
              }
            }
          }
        }
        n244 = local read "Completed"() -> (w608:bool)
        n245 = local read "Exit"() -> (w607:bool)
        n246 = Compound Arithmetic op=OR(w608, w607) -> (w606:bool)
        "No.data" <- w619
      }
      n247 = while {
        tunnel: w414 -> [w471]
        tunnel: w413 -> [_]
        tunnel: w412 -> [_]
        tunnel: [w468] -> w411
        stop <- w469 stop-if-true
        n248 = local read "Output"() -> (w459:dbl[][])
        n249 = local read "No. Y"() -> (w466:i32)
        n250 = call "CursorPosition.vi"("Cursor No."=1.0, "Cursor"="Cursor", "3D Surface Analysis"="3D Surface") -> ("Cursor Y"=w461:dbl)  [unwired: 6 in, 2 out]
        n251 = Dequeue Element(queue=w471, timeout in ms (-1)=3000) -> (queue out=w468:refnum<queue>)  [unwired: 1 in, 3 out]
        n252 = Add(x=w466, y=w461) -> (x+y=w465:dbl)
        n253 = Index Array(array=w459, index (col)=w465) -> (element=→"Feature extraction scan":dbl[])  [unwired: 1 in]
        n254 = call <vilib>:"3D Surface.vi"("z matrix"=w459, "3D graph"="3D Surface") -> ()  [unwired: 8 in, 2 out]
        n255 = local read "Completed"() -> (w467:bool)
        n256 = local read "Exit"() -> (w470:bool)
        n257 = Compound Arithmetic op=OR(w467, w470) -> (w469:bool)
        n258 = Wait Until Next ms Multiple(millisecond multiple=u32 100 ("ms 배수")) -> ()  [unwired: 1 out]
      }
      n259 = Release Queue(queue=w411) -> ()  [unwired: 2 in, 3 out]
      n260 = while {
        stop <- w444 stop-if-true
        n261 = event shown="[0] \"Plot style\", \"ViewMode\": Value Change" {
          selector: _ -> [_ _ _]
          dyn-events: _ -> [_ _ _]
          timeout: _ -> [_ _ _]
          tunnel: [_ w448 _] -> w444
          event "Plot style", "ViewMode": Value Change {
            n262 = event-data() -> ()  [unwired: 1 in, 2 out]
            n263 = local read "3D Surface"() -> (w447:refnum<k7>)
            n264 = property class="CWGraph3D"(reference=w447, "ViewMode"="ViewMode") -> ()  [unwired: 1 in, 2 out]
            n265 = call <vilib>:"Basic Properties.vi"("3D graph"=w447, "plot style"="Plot style") -> ()  [unwired: 12 in, 2 out]
          }
          event "Exit": Value Change {
            n266 = event-data() -> ()  [unwired: 1 in, 1 out]
            n267 = local read "Exit"() -> (w448:bool)
          }
          event "Max", "Min", "ColorMapAutoScale": Value Change {
            n268 = event-data() -> ()  [unwired: 1 in, 5 out]
            n269 = local read "3D Surface"() -> (w449:refnum<k7>)
            n270 = call "Surface_ColorScale.vi"("ColorMapAutoScale"="ColorMapAutoScale", "Min"="Min", "Max"="Max", "3D Surface_"=w449) -> ("Min 2"=w453:dbl, "Max 2"=w452:dbl)  [unwired: 1 in, 2 out]
            n271 = local write "Max"(w452) -> ()
            n272 = local write "Min"(w453) -> ()
          }
        }
      }
      n273 = TDMS Close(8:w419, 11:w420) -> (0:w417:errorcluster)  [unwired: 1 out]
      n274 = call <vilib>:"Simple Error Handler.vi"("error in (no error)"=w417) -> ()  [unwired: 2 in, 7 out]
      n275 = Release Queue(queue=w415) -> ()  [unwired: 2 in, 3 out]
      n276 = while {
        tunnel: w410 -> [w457]
        stop <- w456 stop-if-true
        n277 = call "CSV Save.vi"("Array"=w457, "Save Button"="Save Scan mode") -> ()  [unwired: 9 in, 1 out]
        n278 = Wait Until Next ms Multiple(millisecond multiple=u32 100 ("ms 배수")) -> ()  [unwired: 1 out]
        n279 = local read "Exit"() -> (w456:bool)
      }
    }
    frame "Lift-Off" {
      n280 = while {
        shift-right: [w708] -> _
        shift-left: "2D Array In" -> [w709]
        stop <- w713 stop-if-true
        n281 = call "CSV Open.vi"("2D Array In"=w709, "Open"="Open") -> ("2D Array Out"=w708:dbl[][])  [unwired: 9 in]
        n282 = Delete From Array(array=w708, index (col)=0 ("disabled index (col)")) -> (array with subset deleted=w710:dbl[][])  [unwired: 2 in, 1 out]
        n283 = Subtract(x=w710, y=w708) -> (x-y=w706:dbl[][])
        n284 = Transpose 2D Array(2D array=w706) -> (transposed array=w703:dbl[][])
        n285 = call "Filter_Lowpass - 2D.vi"("Filter"="Filter lf", "Input 2D"=w703, "low cutoff freq: fl"="Low cutoff freq: fl") -> ("Output"=w705:dbl[][])  [unwired: 6 in]
        n286 = Transpose 2D Array(2D array=w705) -> (transposed array=w702:dbl[][])
        n287 = Select(t=w702, s="View Mode", f=w708) -> (s? t:f=→"Hall sensors signal lf":dbl[][])
        n288 = local read "Exit"() -> (w713:bool)
      }
    }
    frame "                    Test mode                   " {
      n289 = while {
        tunnel: w725 -> [w742]
        tunnel: w721 -> [w741]
        tunnel: [w759] -> w723
        tunnel: [w760] -> w724
        shift-right: [w755] -> _
        shift-left: w722 -> [w756]
        tunnel: w722 -> [w754]
        shift-right: [w752] -> _
        shift-left: _ -> [w751]
        tunnel: w720 -> [w750]
        shift-right: [w749] -> _
        shift-left: _ -> [w748]
        shift-right: [w746] -> _
        shift-left: 1 ("Average") -> [w745]
        tunnel: w718 -> [w738]
        tunnel: w717 -> [w737]
        tunnel: w716 -> [w736]
        tunnel: w715 -> [w732]
        shift-right: [w726] -> _
        shift-left: dbl[][] [] -> [w727]
        stop <- w761 stop-if-true
        n290 = First Call?() -> (First Call?: T/F=w743:bool)
        n291 = case shown="True" w743 {
          tunnel: w742 -> [w762 w767]
          tunnel: w741 -> [w763 w766]
          tunnel: [w762 w765] -> w740
          tunnel: [w763 w764] -> w739
          frame False {
          }
          frame True {
            n292 = call <vilib>:"DAQmx Start Task.vi"("task/channels in"=w767, "error in"=w766) -> ("task out"=w765:refnum<k21>, "error out"=w764:errorcluster)  [unwired: 12 in]
          }
        }
        n293 = local read "Pulser Cycles"() -> (w744:i32)
        n294 = call-poly <vilib>:"DAQmx Read.vi"("task/channels in"=w740, "number of samples per channel"=w732, "error in"=w739) -> ("task out"=w760:refnum<k21>, "data"=w730:waveform(dbl)[], "error out"=w759:errorcluster)  [unwired: 10 in]
        n295 = Quotient & Remainder(x=w745, y=w744) -> (x-y*floor(x/y)=w757:i32)  [unwired: 1 out]
        n296 = Equal To 0?(x=w757) -> (x = 0?=w735:bool)
        n297 = Index Array(array=w730, index #1=0 ("index (row)"), index #2=1 ("index")) -> (element #1=w733:waveform(dbl), element #2=w728:waveform(dbl))
        n298 = Unbundle By Name(w733) -> ("Y"=w731:dbl[])
        n299 = Add(x=w731, y=w756) -> (x+y=w753:dbl[])
        n300 = case shown="True" w735 {
          tunnel: w744 -> [_ w801]
          tunnel: w733 -> [_ w795]
          tunnel: w753 -> [w773 w807]
          tunnel: [w773 w806] -> w755
          tunnel: w754 -> [_ w806]
          tunnel: [w772 w804] -> w752
          tunnel: w751 -> [w772 w805]
          tunnel: w750 -> [_ w790]
          tunnel: [w771 w802] -> w749
          tunnel: w748 -> [w771 w803]
          tunnel: [w769 1 ("Average")] -> w746
          tunnel: w745 -> [w770 _]
          tunnel: w738 -> [_ w791]
          tunnel: w737 -> [_ w793]
          tunnel: w736 -> [_ w792]
          tunnel: w728 -> [_ _]
          tunnel: [w768 w784] -> w726
          tunnel: w727 -> [w768 w783]
          frame False {
            n301 = Increment(x=w770) -> (x+1=w769:i32)
          }
          frame True {
            n302 = Divide(x=w807, y=w801) -> (x/y=w774:dbl[])
            "Hall sensors signal" <- w774
            n303 = Bundle By Name(cluster=w795, "Y"=w774) -> (w796:waveform(dbl))
            n304 = xnode "Spectral Measurements"("신호"=w796) -> ("PSD"=w798:cluster{"f0":dbl, "df":dbl, "magnitude":dbl[]})  [unwired: 1 in, 1 out]
            n305 = call "PECT_Feature extraction.vi"("Length T/2"=w790, "Offset"="Offset", "Length"=w791, "Start 2"=w792, "Start 1"=w793, "Pulse signal in"=w774) -> ()  [unwired: 5 in, 1 out]
            n306 = case shown="True" "2 Plots" {
              tunnel: [w815 w821] -> _
              tunnel: w805 -> [_ w820]
              tunnel: [w812 w820] -> w804
              tunnel: w796 -> [w812 w816]
              tunnel: w798 -> [w813 w818]
              tunnel: [w814 w819] -> w797
              tunnel: w803 -> [_ w817]
              tunnel: [w813 w817] -> w802
              frame False {
                n307 = Build Array(w813, w813) -> (w814:cluster{"f0":dbl, "df":dbl, "magnitude":dbl[]}[])
                n308 = Build Array(w812, w812) -> (w815:waveform(dbl)[])
              }
              frame True {
                n309 = Build Array(w817, w818) -> (w819:cluster{"f0":dbl, "df":dbl, "magnitude":dbl[]}[])
                n310 = Build Array(w820, w816) -> (w821:waveform(dbl)[])
              }
            }
            "Power spectral density" <- w797
            n311 = case shown="True" "Add LF" {
              tunnel: w774 -> [_ w811]
              tunnel: [w808 w809] -> w784
              tunnel: w783 -> [w808 w810]
              frame False {
              }
              frame True {
                n312 = Build Array (concatenate)(w810, w811) -> (w809:dbl[][])
              }
            }
            n313 = Subtract(x="End idx", y="Start idx") -> (x-y=w775:i32)
            n314 = Array Subset(array=w774, index="Start idx", length=w775) -> (w778:dbl[])
            n315 = Absolute Value(x=w778) -> (abs(x)=w782:dbl[])
            n316 = Array Size(array=w778) -> (size(s)=w780:i32)
            n317 = Add Array Elements(numeric array=w782) -> (sum=w781:dbl)
            n318 = call "CSV Save.vi"("Array"=w784, "Save Button"="Save LF") -> ()  [unwired: 9 in, 1 out]
            n319 = Divide(x=w781, y=w780) -> (x/y=→"Feature Extraction":dbl)
            n320 = Delete From Array(array=w784, index (col)=0 ("disabled index (col)")) -> (array with subset deleted=w785:dbl[][])  [unwired: 2 in, 1 out]
            n321 = Subtract(x=w785, y=w784) -> (x-y=→"dy":dbl[][])
          }
        }
        n322 = local read "Exit"() -> (w747:bool)
        n323 = Unbundle By Name(w759) -> ("status"=w758:bool)
        n324 = Or(x=w758, y=w747) -> (x .or. y?=w761:bool)
      }
    }
  }
  n325 = VISA Close(VISA resource name=w40, error in (no error)=w39) -> (error out=w37:errorcluster)
  n326 = VISA Close(VISA resource name=w41, error in (no error)=w42) -> (error out=w38:errorcluster)
  n327 = call <vilib>:"Simple Error Handler.vi"("error in (no error)"=w37) -> ()  [unwired: 4 in, 5 out]
  n328 = call <vilib>:"Simple Error Handler.vi"("error in (no error)"=w38) -> ()  [unwired: 4 in, 5 out]
  n329 = while {
    shift-right: [w851] -> _
    shift-left: T1."No Scan" -> [w856]
    shift-right: [w847] -> _
    shift-left: 0.0 ("Current  Position (mm)") -> [w855]
    shift-right: [w848] -> _
    shift-left: 0.0 ("Current  Position (mm)") -> [w854]
    shift-right: [w846] -> _
    shift-left: 0.0 ("Current  Position (mm)") -> [w853]
    shift-right: [w845] -> _
    shift-left: 0.0 ("Current  Position (mm)") -> [w852]
    tunnel: w27 -> [w850]
    tunnel: w26 -> [w837]
    tunnel: w29 -> [w849]
    tunnel: w28 -> [w836]
    tunnel: [w844] -> _
    tunnel: [w842] -> w35
    tunnel: [w843] -> _
    tunnel: [w841] -> w36
    shift-right: [w834] -> _
    shift-left: 0.0 ("Current  Position (mm)") -> [w833]
    stop <- w838 stop-if-true
    n330 = case shown="\"Wait X\"" w856 {
      selector: w856 -> [w875 _ _ _ _]
      tunnel: w855 -> [w868 w935 w957 w1021 w1061]
      tunnel: w854 -> [w869 w934 w963 w1020 w1060]
      tunnel: w853 -> [_ w933 w980 w1001 w1044]
      tunnel: w852 -> [_ w932 w981 w1019 w1042]
      tunnel: [w874 T1."Wait X" w959 w1012 w1046] -> w851
      tunnel: w850 -> [w873 w927 w976 w1010 w1055]
      tunnel: w837 -> [w872 w928 w977 w1011 w1056]
      tunnel: w849 -> [w871 w929 w969 w1006 w1058]
      tunnel: w836 -> [w870 w930 w970 w1007 w1057]
      tunnel: [w861 w934 w963 w1020 w1060] -> w848
      tunnel: [w860 w935 w960 w1021 w1061] -> w847
      tunnel: [w863 w933 w980 w1001 w1059] -> w846
      tunnel: [w862 w932 w981 w1019 w1042] -> w845
      tunnel: [w867 w921 w974 w1009 w1053] -> w844
      tunnel: [w866 w920 w972 w1008 w1051] -> w842
      tunnel: [w865 w919 w978 w1004 w1049] -> w843
      tunnel: [w864 w918 w979 w1005 w1047] -> w841
      tunnel: w837 -> [_ _ _ _ _]
      tunnel: [w859 w917 w950 w999 w1038] -> w834
      tunnel: w833 -> [w858 w917 w956 w999 w1038]
      frame "No Scan", Default {
        n331 = local read "Scan"() -> (w857:bool)
        n332 = case shown="True" w857 {
          tunnel: w875 -> [w883 _]
          tunnel: [w883 w894] -> w874
          tunnel: w873 -> [w880 w892]
          tunnel: w872 -> [w881 w891]
          tunnel: w871 -> [w878 w890]
          tunnel: w870 -> [w879 w889]
          tunnel: w869 -> [w877 _]
          tunnel: w868 -> [w882 _]
          tunnel: [w882 w888] -> w860
          tunnel: [w881 w898] -> w867
          tunnel: [w880 w897] -> w866
          tunnel: [w879 w896] -> w865
          tunnel: [w878 w895] -> w864
          tunnel: [w877 w893] -> w863
          tunnel: [w876 w888] -> w859
          tunnel: w858 -> [w876 _]
          frame False {
          }
          frame True {
            n333 = flat-sequence {
              tunnel: w889 -> [w899]
              tunnel: w890 -> [w900]
              tunnel: w891 -> [w901]
              tunnel: w892 -> [w902]
              tunnel: [w902] -> w887
              tunnel: [w901] -> w886
              tunnel: [w900] -> w885
              tunnel: [w899] -> w884
              tunnel: [w916] -> w898
              tunnel: [w915] -> w897
              tunnel: [w914] -> w896
              tunnel: [w913] -> w895
              tunnel: [T1."Move X"] -> w894
              tunnel: [w911] -> w893
              tunnel: [w904] -> w888
              tunnel: w887 -> [w910]
              tunnel: w886 -> [w909]
              tunnel: w885 -> [w908]
              tunnel: w884 -> [w907]
              frame #0 {
              }
              frame #1 {
                n334 = local write "Direction (+)"("+" ("Direction (+)")) -> ()
                n335 = local write "Numeric"(0.0 ("Numeric")) -> ()
                n336 = local read "Travel per Pulse (mm)"() -> (w906:dbl)
                n337 = call "Autonics_GetPos.vi"("error in (no error)"=w910, "Travel per Pulse (mm)"=w906, "VISA resource name"=w909) -> ("error out"=w915:errorcluster, "Current  Position (mm)"=w904:dbl, "VISA resource name out"=w916:refnum<visa-resource-name>)  [unwired: 6 in]
                "Start Pos Y" <- w904
                n338 = call "Autonics_GetPos.vi"("error in (no error)"=w908, "Travel per Pulse (mm)"=w906, "VISA resource name"=w907) -> ("error out"=w913:errorcluster, "Current  Position (mm)"=w911:dbl, "VISA resource name out"=w914:refnum<visa-resource-name>)  [unwired: 6 in]
                "Start Pos X" <- w911
                n339 = local write "Cur. Pos X"(w904) -> ()
                n340 = local write "Cur. Pos Y"(w911) -> ()
              }
            }
          }
        }
        n341 = local read "X - length"() -> (w861:dbl)
        n342 = local read "Step Y"() -> (w862:dbl)
      }
      frame "Move X" {
        n343 = local read "Travel per Pulse (mm)"() -> (w922:dbl)
        n344 = local read "X - length"() -> (w923:dbl)
        n345 = call "Autonics_Move.vi"("Direction (+)"="Direction (+)", "error in (no error)"=w927, "Travel per Pulse (mm)"=w922, "Move Distance (mm)"=w923, "VISA resource name"=w928) -> ("error out"=w925:errorcluster, "VISA resource name out"=w926:refnum<visa-resource-name>)  [unwired: 5 in]
        n346 = flat-sequence {
          tunnel: [w940] -> w921
          tunnel: w926 -> [w940]
          tunnel: [w939] -> w920
          tunnel: w925 -> [w939]
          tunnel: [w937] -> w919
          tunnel: w930 -> [w937]
          tunnel: [w936] -> w918
          tunnel: w929 -> [w936]
          frame #0 {
            n347 = Wait (ms)(milliseconds to wait=u32 100) -> ()  [unwired: 1 out]
          }
        }
      }
      frame "Wait X" {
        n348 = local read "Travel per Pulse (mm)"() -> (w967:dbl)
        n349 = call "Autonics_GetPos.vi"("error in (no error)"=w969, "Travel per Pulse (mm)"=w967, "VISA resource name"=w970) -> ("error out"=w968:errorcluster, "Current  Position (mm)"=w966:dbl, "VISA resource name out"=w971:refnum<visa-resource-name>)  [unwired: 6 in]
        n350 = call "Autonics_GetPos.vi"("error in (no error)"=w976, "Travel per Pulse (mm)"=w967, "VISA resource name"=w977) -> ("error out"=w973:errorcluster, "Current  Position (mm)"=w948:dbl, "VISA resource name out"=w975:refnum<visa-resource-name>)  [unwired: 6 in]
        n351 = local read "Direction (+)"() -> (w943:string)
        n352 = local write "Cur. Pos Y"(w966) -> ()
        n353 = Equal?(x=w943, y="-") -> (x = y?=w941:bool)
        n354 = local read "Step X"() -> (w953:dbl)
        n355 = local write "Cur. Pos X"(w948) -> ()
        n356 = Subtract(x=w948, y=w956) -> (x-y=w955:dbl)
        n357 = Absolute Value(x=w963) -> (abs(x)=w965:dbl)
        n358 = Absolute Value(x=w955) -> (abs(x)=w954:dbl)
        n359 = Subtract(x=w948, y=w957) -> (x-y=w964:dbl)
        n360 = Greater Or Equal?(x=w954, y=w953) -> (x >= y?=w949:bool)
        n361 = Quotient & Remainder(x=w948, y=w953) -> (floor(x/y)=w945:dbl)  [unwired: 1 out]
        n362 = Absolute Value(x=w964) -> (abs(x)=w958:dbl)
        n363 = Subtract(x=w958, y=w965) -> (x-y=w961:dbl)
        n364 = case shown="True" w949 {
          selector: w949 -> [_ w982]
          frame False {
          }
          frame True {
            n365 = local read "Numeric"() -> (w984:dbl)
            n366 = Increment(x=w984) -> (x+1=→"Numeric":dbl)
            "Acquire" <- w982
          }
        }
        n367 = Increment(x=w945) -> (x+1=w946:dbl)
        n368 = call "Convert Double Precision.vi"("Input"=w961) -> ("Output"=w962:dbl)  [unwired: 10 in]
        n369 = Select(t=w946, s=w941, f=w945) -> (s? t:f=w944:dbl)
        n370 = Multiply(x=w944, y=w953) -> (x*y=w952:dbl)
        n371 = Select(t=w952, s=w949, f=w956) -> (s? t:f=w951:dbl)
        n372 = Greater Or Equal To 0?(x=w962) -> (x >= 0?=w947:bool)
        n373 = Select(t=w948, s=w947, f=w951) -> (s? t:f=w950:dbl)
        n374 = case shown="True" w947 {
          tunnel: [w987 w998] -> w979
          tunnel: w968 -> [w987 w998]
          tunnel: [w988 w997] -> w978
          tunnel: w971 -> [w988 w997]
          tunnel: [w990 w996] -> w974
          tunnel: w975 -> [w990 w996]
          tunnel: [w989 w995] -> w972
          tunnel: w973 -> [w989 w995]
          tunnel: [w986 w994] -> w960
          tunnel: w957 -> [w986 _]
          tunnel: [T1."Wait X" T1."Move Y"] -> w959
          frame False {
          }
          frame True {
            n375 = local read "Cur. Pos X"() -> (w994:dbl)
            n376 = local write "Numeric"(0.0 ("Numeric")) -> ()
            n377 = Wait (ms)(milliseconds to wait=u32 1000) -> ()  [unwired: 1 out]
          }
        }
        "Current  Position (mm)" <- w956
      }
      frame "Move Y" {
        n378 = local read "Step Y"() -> (w1015:dbl)
        n379 = local read "Y - length"() -> (w1000:dbl)
        n380 = local read "Start Pos Y"() -> (w1002:dbl)
        n381 = Subtract(x=w1000, y=w1015) -> ()  [unwired: 1 out]
        n382 = Subtract(x=w1002, y=w1001) -> (x-y=w1018:dbl)
        n383 = Absolute Value(x=w1000) -> (abs(x)=w1016:dbl)
        n384 = Absolute Value(x=w1018) -> (abs(x)=w1017:dbl)
        n385 = Subtract(x=w1017, y=w1016) -> (x-y=w1014:dbl)
        n386 = call "Convert Double Precision.vi"("Input"=w1014) -> ("Output"=w1013:dbl)  [unwired: 10 in]
        n387 = Greater Or Equal To 0?(x=w1013) -> (x >= 0?=w1003:bool)
        n388 = case shown="True" w1003 {
          tunnel: [T1."Wait Y" T1."No Scan"] -> w1012
          tunnel: w1011 -> [w1029 w1035]
          tunnel: [w1030 w1034] -> w1008
          tunnel: w1010 -> [w1030 w1034]
          tunnel: [w1029 w1035] -> w1009
          tunnel: w1007 -> [w1023 w1033]
          tunnel: w1006 -> [w1027 w1032]
          tunnel: [w1028 w1032] -> w1005
          tunnel: [w1022 w1033] -> w1004
          frame False {
            n389 = local read "Step Y"() -> (w1026:dbl)
            n390 = local read "Travel per Pulse (mm)"() -> (w1024:dbl)
            n391 = call "Autonics_Move.vi"("Direction (+)"="+" ("Direction (+) 2"), "error in (no error)"=w1027, "Travel per Pulse (mm)"=w1024, "Move Distance (mm)"=w1026, "VISA resource name"=w1023) -> ("error out"=w1028:errorcluster, "VISA resource name out"=w1022:refnum<visa-resource-name>)  [unwired: 5 in]
          }
          frame True {
            n392 = local write "Scan"(FALSE) -> ()
          }
        }
      }
      frame "Wait Y" {
        n393 = local read "Travel per Pulse (mm)"() -> (w1039:dbl)
        n394 = call "Autonics_GetPos.vi"("error in (no error)"=w1058, "Travel per Pulse (mm)"=w1039, "VISA resource name"=w1057) -> ("error out"=w1048:errorcluster, "Current  Position (mm)"=w1043:dbl, "VISA resource name out"=w1050:refnum<visa-resource-name>)  [unwired: 6 in]
        n395 = call "Autonics_GetPos.vi"("error in (no error)"=w1055, "Travel per Pulse (mm)"=w1039, "VISA resource name"=w1056) -> ("error out"=w1052:errorcluster, "Current  Position (mm)"=w1045:dbl, "VISA resource name out"=w1054:refnum<visa-resource-name>)  [unwired: 6 in]
        n396 = Subtract(x=w1043, y=w1044) -> (x-y=w1063:dbl)
        n397 = Absolute Value(x=w1042) -> (abs(x)=w1065:dbl)
        n398 = Absolute Value(x=w1063) -> (abs(x)=w1064:dbl)
        n399 = Subtract(x=w1064, y=w1065) -> (x-y=w1062:dbl)
        n400 = local write "Cur. Pos X"(w1045) -> ()
        n401 = local write "Cur. Pos Y"(w1043) -> ()
        n402 = call "Convert Double Precision.vi"("Input"=w1062) -> ("Output"=w1041:dbl)  [unwired: 10 in]
        n403 = Greater Or Equal To 0?(x=w1041) -> (x >= 0?=w1040:bool)
        n404 = case shown="True" w1040 {
          tunnel: w1044 -> [w1071 _]
          tunnel: [w1071 w1084] -> w1059
          tunnel: w1054 -> [w1070 w1082]
          tunnel: [w1070 w1082] -> w1053
          tunnel: [w1069 w1081] -> w1051
          tunnel: w1052 -> [w1069 w1081]
          tunnel: [w1068 w1080] -> w1049
          tunnel: w1050 -> [w1068 w1080]
          tunnel: [w1067 w1079] -> w1047
          tunnel: w1048 -> [w1067 w1079]
          tunnel: [T1."Wait Y" T1."Move X"] -> w1046
          frame False {
          }
          frame True {
            n405 = local read "Direction (+)"() -> (w1078:string)
            n406 = local read "Cur. Pos Y"() -> (w1084:dbl)
            n407 = Equal?(x=w1078, y="+") -> (x = y?=w1076:bool)
            n408 = Select(t="-", s=w1076, f="+") -> (s? t:f=w1075:string)
            n409 = local write "Direction (+)"(w1075) -> ()
            n410 = Wait (ms)(milliseconds to wait=u32 1000) -> ()  [unwired: 1 out]
          }
        }
      }
    }
    n411 = Wait Until Next ms Multiple(millisecond multiple=u32 100 ("milliseconds to wait")) -> ()  [unwired: 1 out]
    n412 = local read "Completed"() -> (w832:bool)
    n413 = local read "Exit"() -> (w831:bool)
    n414 = Unbundle By Name(w841) -> ("status"=w839:bool)
    n415 = Unbundle By Name(w842) -> ("status"=w840:bool)
    n416 = Compound Arithmetic op=OR(w832, w831, w840, w839) -> (w838:bool)
    "Enum" <- w856
  }
  n417 = call <vilib>:"DAQmx Clear Task.vi"("task in"=w90, "error in"=w89) -> ("error out"=w96:errorcluster)  [unwired: 13 in]
  n418 = call <vilib>:"Simple Error Handler.vi"("error in (no error)"=w96) -> ()  [unwired: 4 in, 5 out]
  n419 = call <vilib>:"Simple Error Handler.vi"("error in (no error)"=w35) -> ()  [unwired: 4 in, 5 out]
  n420 = call <vilib>:"Simple Error Handler.vi"("error in (no error)"=w36) -> ()  [unwired: 4 in, 5 out]
  n421 = call <vilib>:"Simple Error Handler.vi"() -> ()  [unwired: 5 in, 5 out]
